vi "EditorEinfachCRIOalteMethoden-15-07-17.vi"() -> ()   [LabVIEW 2017]
panel:
  out "Methoden":T1(array[cluster])
  in  "Tab Control":T2(tab)
  in  "Dateiordner Housekeeping":path=path "C:/Users/Atmos/Desktop/Johnny"
  in  "Dateiname Housekeeping":string
  in  "DateiordnerECD1":path
  in  "DateinameECD1":string
  in  "DateiordnerECD2":path
  in  "DateinameECD2":string
  in  "Modul1/AI sicherer Bereich":dbl[][](array[numeric])=[[0.0, 0.0, 0.0, 0.0, 0.0, 0.0, 0.0, 0.0, 0.0, 0.0, 0.0, 0.0, 0.0, 0.0, 0.0, 0.0, 0.0, 0.0, 0.0, 0.0, 0.0, 0.0, 0.0, 0.0, 0.0, 0.0, 0.0, 0.0, 0.0, 0.0, 0.0, 0.0]]
  in  "Modul1/AIsNamen":string[](array[string])
  in  "Modul1/AI koeff":dbl[][](array[numeric])=[[0.0, 0.0, 0.0, 0.0, 0.0, 0.0, 0.0, 0.0, 0.0, 0.0, 0.0, 0.0, 0.0, 0.0, 0.0, 0.0, 0.0, 0.0, 0.0, 0.0, 0.0, 0.0, 0.0, 0.0, 0.0, 0.0, 0.0, 0.0, 0.0, 0.0, 0.0, 0.0]]
  in  "AIsNamenZurücksetzen":bool
  in  "Modul2/AIsNamen":string[](array[string])
  in  "Modul2/AI koeff":dbl[][](array[numeric])=[[0.0, 0.0, 0.0, 0.0, 0.0, 0.0, 0.0, 0.0, 0.0, 0.0, 0.0, 0.0, 0.0, 0.0, 0.0, 0.0, 0.0, 0.0, 0.0, 0.0, 0.0, 0.0, 0.0, 0.0, 0.0, 0.0, 0.0, 0.0, 0.0, 0.0, 0.0, 0.0]]
  in  "Modul2/AI sicherer Bereich":dbl[][](array[numeric])=[[0.0, 0.0, 0.0, 0.0, 0.0, 0.0, 0.0, 0.0, 0.0, 0.0, 0.0, 0.0, 0.0, 0.0, 0.0, 0.0, 0.0, 0.0, 0.0, 0.0, 0.0, 0.0, 0.0, 0.0, 0.0, 0.0, 0.0, 0.0, 0.0, 0.0, 0.0, 0.0]]
  in  "Modul3/AIsNamen":string[](array[string])
  in  "Modul3/AI koeff":dbl[][](array[numeric])=[[0.0, 0.0, 0.0, 0.0, 0.0, 0.0, 0.0, 0.0, 0.0, 0.0, 0.0, 0.0, 0.0, 0.0, 0.0, 0.0, 0.0, 0.0, 0.0, 0.0, 0.0, 0.0, 0.0, 0.0, 0.0, 0.0, 0.0, 0.0, 0.0, 0.0, 0.0, 0.0]]
  in  "Modul3/AI sicherer Bereich":dbl[][](array[numeric])=[[0.0, 0.0, 0.0, 0.0, 0.0, 0.0, 0.0, 0.0, 0.0, 0.0, 0.0, 0.0, 0.0, 0.0, 0.0, 0.0, 0.0, 0.0, 0.0, 0.0, 0.0, 0.0, 0.0, 0.0, 0.0, 0.0, 0.0, 0.0, 0.0, 0.0, 0.0, 0.0]]
  in  "Traps/MachsKoeff R(U)":dbl[][](array[numeric])=[[0.0, 0.0, 0.0, 0.0, 0.0, 0.0, 0.0, 0.0, 0.0, 0.0, 0.0, 0.0, 0.0, 0.0, 0.0, 0.0, 0.0, 0.0, 0.0, 0.0, 0.0, 0.0, 0.0, 0.0, 0.0, 0.0, 0.0, 0.0, 0.0, 0.0, 0.0, 0.0]]
  out "Schnelle Heizungen":string[](array[string])
  in  "Traps/MachsKoeff T(R)":dbl[][](array[numeric])=[[0.0, 0.0, 0.0, 0.0, 0.0, 0.0, 0.0, 0.0, 0.0, 0.0, 0.0, 0.0, 0.0, 0.0, 0.0, 0.0, 0.0, 0.0, 0.0, 0.0, 0.0, 0.0, 0.0, 0.0, 0.0, 0.0, 0.0, 0.0, 0.0, 0.0, 0.0, 0.0]]
  in  "Traps/Machs sicherer Bereich":dbl[][](array[numeric])=[[0.0, 0.0, 0.0, 0.0, 0.0, 0.0, 0.0, 0.0, 0.0, 0.0, 0.0, 0.0, 0.0, 0.0, 0.0, 0.0, 0.0, 0.0, 0.0, 0.0, 0.0, 0.0, 0.0, 0.0, 0.0, 0.0, 0.0, 0.0, 0.0, 0.0, 0.0, 0.0]]
  in  "LangsameHeizungen":string[](array[string])
  in  "ModuleLH":i32[](array[numeric]) min=1 max=3 step=1
  in  "AIsLH":i32[](array[numeric]) min=0 max=31 step=1
  in  "LHGruppe":bool[](array[boolean])
  in  "DIOsMod0Name":string[](array[string])
  in  "DIOsMod0Nr":i32[](array[numeric]) min=0 max=63 step=1
  in  "DIOsMod1Name":string[](array[string])
  in  "DIOsMod1Nr":i32[](array[numeric]) min=0 max=63 step=1
  in  "DIOsMod2AName":string[](array[string])
  in  "DIOsMod2ANr":i32[](array[numeric]) min=0 max=63 step=1
  in  "DIOsMod2BName":string[](array[string])
  in  "DIOsMod2BNr":i32[](array[numeric]) min=0 max=63 step=1
  out "AnzahlRegler/Modul":i32[](array[numeric])
  in  "Regler für den Probenfluß":i32
  in  "ReglerNameMod0":string[](array[string])
  in  "ReglerNameMod1":string[](array[string])
  in  "ReglerNameMod2A":string[](array[string])
  in  "ReglerNameMod2B":string[](array[string])
  in  "MWabfragenMod0":string[](array[string])=[":060F0401210120", ":06100401210120", ":06110401210120"]
  in  "MWabfragenMod1":string[](array[string])=[":060F0401210120", ":06100401210120", ":06110401210120"]
  in  "MWabfragenMod2A":string[](array[string])=[":060F0401210120", ":06100401210120", ":06110401210120"]
  in  "MWabfragenMod2B":string[](array[string])=[":060F0401210120", ":06100401210120", ":06110401210120"]
  in  "SPvorgebenMod0":string[](array[string])=[":060F020121", ":0610020121", ":0611020121"]
  in  "SPvorgebenMod1":string[](array[string])=[":060F020121", ":0610020121", ":0611020121"]
  in  "SPvorgebenMod2A":string[](array[string])=[":060F020121", ":0610020121", ":0611020121"]
  in  "SPvorgebenMod2B":string[](array[string])=[":060F020121", ":0610020121", ":0611020121"]
  in  "FaktorMod0":dbl[](array[numeric])=[9.375e-05, 9.375e-05, 9.375e-05]
  in  "FaktorMod1":dbl[](array[numeric])=[9.375e-05, 9.375e-05, 9.375e-05]
  in  "FaktorMod2A":dbl[](array[numeric])=[9.375e-05, 9.375e-05, 9.375e-05]
  in  "FaktorMod2B":dbl[](array[numeric])=[9.375e-05, 9.375e-05, 9.375e-05]
  in  "MWAntwortMod0":string[](array[string])=[":060F020121", ":0610020121", ":0611020121"]
  in  "MWAntwortMod1":string[](array[string])=[":060F020121", ":0610020121", ":0611020121"]
  in  "MWAntwortMod2A":string[](array[string])=[":060F020121", ":0610020121", ":0611020121"]
  in  "MWAntwortMod2B":string[](array[string])=[":060F020121", ":0610020121", ":0611020121"]
  in  "ReglerMod0 sicherer Bereich":dbl[][](array[numeric])=[[9.375e-05, 9.375e-05, 9.375e-05]]
  in  "ReglerMod1 sicherer Bereich":dbl[][](array[numeric])=[[9.375e-05, 9.375e-05, 9.375e-05]]
  in  "ReglerMod2A sicherer Bereich":dbl[][](array[numeric])=[[9.375e-05, 9.375e-05, 9.375e-05]]
  in  "ReglerMod2B sicherer Bereich":dbl[][](array[numeric])=[[9.375e-05, 9.375e-05, 9.375e-05]]
  in  "Metavariablen grüner Bereich":dbl[][](array[numeric])=[[0.0, 0.0, 0.0, 0.0, 0.0, 0.0, 0.0, 0.0, 0.0, 0.0, 0.0, 0.0, 0.0, 0.0, 0.0, 0.0, 0.0, 0.0, 0.0, 0.0, 0.0, 0.0, 0.0, 0.0, 0.0, 0.0, 0.0, 0.0, 0.0, 0.0, 0.0, 0.0]]
  in  "Metavariablen":string[](array[string])
  in  "Startmethode":i32=1
  in  "MethodeLöschen":bool
  in  "MethodeDuplizieren":bool
  in  "T_MainMach2":dbl[](array[numeric])
  in  "t_MainMach2":dbl[](array[numeric])
  in  "T_MainMach1":dbl[](array[numeric])
  in  "t_MainMach1":dbl[](array[numeric])
  in  "EinstellungenSpeichern":bool
  out "LangsameHeizungen":string[](array[string])
  in  "AllesSpeichern":bool
  in  "Methodenname":string
  in  "Int.Stop2":dbl
  in  "Int.Start2":dbl
  in  "Int.Stop1":dbl
  in  "Int.Start1":dbl
  in  "ZeitpktMS-2":dbl
  in  "ZeitpktMS-1":dbl
  in  "SPMPV":i32[](array[numeric])
  in  "ZeitpunkteMPV":dbl[](array[numeric])
  in  "Wert2":dbl
  in  "Vergleichsoperator2":dbl(ring) items=["<", "<=", "=", ">=", ">", "=/="]
  in  "AbfragbareVariablen2":dbl(ring) items=["T1-Trap1 [°C]", "T1-Trap2 [°C]", "T1-StirlingKühlkopf [°C]", "T1-PreCol1 [°C]", "T1-PreCol2 [°C]", "T1-MainCol1a [°C]", "T1-MainCol1b [°C]", "T1-MainCol2a [°C]", "T1-MainCol2b [°C]", "T1-Bronkhorst1a [°C]", "T1-Bronkhorst1b [°C]", "T1-Bronkhorst2a [°C]", "T1-Bronkhorst2b [°C]", "T1-2Pos1B [°C]", "T1-Spare9", "T1-2Pos1A [°C]", "T1-Spare10", "T1-TurboPump [°C]", "T1-StirlingPlatine [°C]", "T1-Spare5", "T1-Spare6", "T1-Spare7", "T1-Spare8", "F1-MFM1", "F1-MFM0D [mL]", "P1-HeliumHP [bara]", "P1-HeliumLP [bara]", "P1-PumpVordruck [mbara]", "TurboSpeed", "I1-MS-AC [A]", "I1-Trap1 [A]", "I1-Trap2 [A]", "T2-ECD1a", "T2-ECD1b", "T2-ECD2a", "T2-ECD2b", "T2-Col1a", "T2-Col1b", "T2-Col2a", "T2-Col2b", "T2-Spare1", "T2-Spare2", "T2-Oven_a", "T2-Oven_b", "T2-Spare3", "T2-Spare4", "T2-Spare5", "F2-MFM0", "F2-MFM2A", "F2-MFM2B", "P2-N2O_HP", "P2-N2O_LP", "P2-CO2_HP", "P2-CO2_LP", "AI-Spare1", "FL-MFM1000mL", "AI-Spare3", "AI-Spare4", "StirlingAlarm", "StirlingEmerg.", "AI-Spare7", "AI-Spare8", "AI-Spare9", "FL-MFM30mL", "T0-DC/DC5", "I0-24V_M0", "I0-48V_M1", "I0-24V_M1", "I0-28V_M2", "T0-Spare3", "T0-Spare2", "T0-Spare4", "T0-DC/DC7", "I0-20V_Laptop", "I0-28V_M1", "I0-24V_M2", "I0-12V_Licor", "T0-Spare1", "T0-Drier", "T0-Spare5", "F0-MFM0A [L]", "TL-Licor_a", "P0-Span-HP", "P0-spare1", "P0-Stickstoff-LP", "P0-Helium-LP", "P0-Cal-HP", "P0-P9Tavco[bar]", "F0-MFM0B [L]", "TL-Licor_b", "P0-Span-LP", "P0-spare2", "P0-Stickstoff-HP", "P0-Helium-HP", "P0-Cal-LP", "F0-MFM3", "T-Trap1", "T-Trap2", "T-PreMach1", "T-PreMach2", "T-MainMach1", "T-MainMach2", "PrC0 [bara]", "PrC0-Licor [bara]", "PrC1-Säule1 [bara]", "PrC1-Säule2 [bara]", "MFC1-Sample [ml/min]", "PrC1-BackFlush1 [bara]", "PrC1-BackFlush2 [bara]", "MFC1-Reaktant [l/min]", "MFC2A[ml/min]", "MFC2B[ml/min]", "MFC2C[ul/min]", "PrC2A[bara]", "MFC2D[ml/min]", "MFC2E[ml/min]", "PrC2B[bara]", "Gesamte Zeit", "Methodenzeit", "Zykluszeit Mod0", "Zykluszeit Mod1", "Zykluszeit Mod2A", "Zykluszeit Mod2B", "PositionMPV", "OverflowB", "OverflowA", "StirlingAlarmAlarm!"]
  in  "Dateien fürs MS schicken?":bool
  in  "Zwangsbedingungen":dbl[][](array[numeric])
  out "ZwangsBedingungen":string[][](array[string])
  in  "löschen":bool
  in  "Bedingung Nr. X":i32
  in  "Bedingung übernehmen":bool
  in  "Ausgangswert":dbl
  in  "BedienbareVariablen":dbl(ring) items=["D0-48V_M1", "D0-28V_M1", "D0-Pump2", "DL-LiCalS1H", "D-Spare2", "D-Spare4", "D0-28V_M2", "D0-Pump1", "D0-S01/EV1", "DL-Licor", "D0-EV3", "D0-EV2", "D1-StopMS", "D1-StartMS", "D1-TrapEvac1", "D1-TrapEvac2", "D1-2Pos1A", "D1-2Pos1B", "D1-TurboPump", "D1-PrePump", "D1-VacPump1", "D1-VacPump2", "D1-Stirling", "D1-P_MS", "D1-S1B(7)", "D1-S1A(6)", "D1-S1G", "D1-Fan3", "D1-LüfterMach1", "D1-LüfterMach2", "D1-MS-Power", "D2-SpülflußA", "D2-2Pos2A", "D2-Probe2A", "D2-ECD1HeaterOff", "D2-Fan1", "D2-Fan2", "D2-Spülfluß2B", "D2-2Pos2B", "D2-Probe2B", "D2-ECD2HeaterOff", "Heizen?Trap1", "Heizen?Trap2", "Heizen?PreMach1", "Heizen?PreMach2", "Heizen?MainMach1", "Heizen?MainMach2", "Methodennummer", "STOPP!!!", "H1-Valve1B heizen?", "H1-Bronkhorst1 heizen?", "H1-Bronkhorst2 heizen?", "H1-Valve1A heizen?", "H0-Drier heizen?", "HL-Licor heizen?", "H2-ECD2 heizen?", "H2-Oven heizen?", "H2-Spare1 heizen?", "H2-Col2 heizen?", "H2-Col1 heizen?", "H2-ECD1 heizen?", "PrC0 [bara]", "PrC0-Licor [bara]", "PrC1-Säule1 [bara]", "PrC1-Säule2 [bara]", "MFC1-Sample [ml/min]", "PrC1-BackFlush1 [bara]", "PrC1-BackFlush2 [bara]", "MFC1-Reaktant [l/min]", "MFC2A[ml/min]", "MFC2B[ml/min]", "MFC2C[ul/min]", "PrC2A[bara]", "MFC2D[ml/min]", "MFC2E[ml/min]", "PrC2B[bara]", "PositionMPV", "OverflowB", "OverflowA", "StirlingAlarmAlarm!"]
  in  "Wert1":dbl
  in  "Vergleichsoperator1":dbl(ring) items=["<", "<=", "=", ">=", ">", "=/="]
  in  "AbfragbareVariablen1":dbl(ring) items=["T1-Trap1 [°C]", "T1-Trap2 [°C]", "T1-StirlingKühlkopf [°C]", "T1-PreCol1 [°C]", "T1-PreCol2 [°C]", "T1-MainCol1a [°C]", "T1-MainCol1b [°C]", "T1-MainCol2a [°C]", "T1-MainCol2b [°C]", "T1-Bronkhorst1a [°C]", "T1-Bronkhorst1b [°C]", "T1-Bronkhorst2a [°C]", "T1-Bronkhorst2b [°C]", "T1-2Pos1B [°C]", "T1-Spare9", "T1-2Pos1A [°C]", "T1-Spare10", "T1-TurboPump [°C]", "T1-StirlingPlatine [°C]", "T1-Spare5", "T1-Spare6", "T1-Spare7", "T1-Spare8", "F1-MFM1", "F1-MFM0D [mL]", "P1-HeliumHP [bara]", "P1-HeliumLP [bara]", "P1-PumpVordruck [mbara]", "TurboSpeed", "I1-MS-AC [A]", "I1-Trap1 [A]", "I1-Trap2 [A]", "T2-ECD1a", "T2-ECD1b", "T2-ECD2a", "T2-ECD2b", "T2-Col1a", "T2-Col1b", "T2-Col2a", "T2-Col2b", "T2-Spare1", "T2-Spare2", "T2-Oven_a", "T2-Oven_b", "T2-Spare3", "T2-Spare4", "T2-Spare5", "F2-MFM0", "F2-MFM2A", "F2-MFM2B", "P2-N2O_HP", "P2-N2O_LP", "P2-CO2_HP", "P2-CO2_LP", "AI-Spare1", "FL-MFM1000mL", "AI-Spare3", "AI-Spare4", "StirlingAlarm", "StirlingEmerg.", "AI-Spare7", "AI-Spare8", "AI-Spare9", "FL-MFM30mL", "T0-DC/DC5", "I0-24V_M0", "I0-48V_M1", "I0-24V_M1", "I0-28V_M2", "T0-Spare3", "T0-Spare2", "T0-Spare4", "T0-DC/DC7", "I0-20V_Laptop", "I0-28V_M1", "I0-24V_M2", "I0-12V_Licor", "T0-Spare1", "T0-Drier", "T0-Spare5", "F0-MFM0A [L]", "TL-Licor_a", "P0-Span-HP", "P0-spare1", "P0-Stickstoff-LP", "P0-Helium-LP", "P0-Cal-HP", "P0-P9Tavco[bar]", "F0-MFM0B [L]", "TL-Licor_b", "P0-Span-LP", "P0-spare2", "P0-Stickstoff-HP", "P0-Helium-HP", "P0-Cal-LP", "F0-MFM3", "T-Trap1", "T-Trap2", "T-PreMach1", "T-PreMach2", "T-MainMach1", "T-MainMach2", "PrC0 [bara]", "PrC0-Licor [bara]", "PrC1-Säule1 [bara]", "PrC1-Säule2 [bara]", "MFC1-Sample [ml/min]", "PrC1-BackFlush1 [bara]", "PrC1-BackFlush2 [bara]", "MFC1-Reaktant [l/min]", "MFC2A[ml/min]", "MFC2B[ml/min]", "MFC2C[ul/min]", "PrC2A[bara]", "MFC2D[ml/min]", "MFC2E[ml/min]", "PrC2B[bara]", "Gesamte Zeit", "Methodenzeit", "Zykluszeit Mod0", "Zykluszeit Mod1", "Zykluszeit Mod2A", "Zykluszeit Mod2B", "PositionMPV", "OverflowB", "OverflowA", "StirlingAlarmAlarm!"]
  in  "Methode Nummer":i32
  in  "MethodeLaden":bool
  in  "EditorBeenden":bool
  in  "PIDs für \"träge\" Heizungen":T3(array[cluster])
  in  "T_PreMach2":dbl[](array[numeric])
  in  "t_PreMach2":dbl[](array[numeric])
  in  "T_PreMach1":dbl[](array[numeric])
  in  "t_PreMach1":dbl[](array[numeric])
  in  "SHSetpoints":dbl[][](array[numeric])
  in  "ZeitpktFPGAFixp":dbl[](array[numeric])
  in  "FPGAPID":T4(array[cluster])
  in  "ZeitpktFPGAPID":dbl[](array[numeric])
  in  "FPGABoolesch":bool[][](array[boolean])
  in  "ZPktFPGABoolesch":dbl[](array[numeric])
  in  "LHHeizen?":bool[](array[boolean])
  in  "LHSetpoints":dbl[](array[numeric])
  out "HorstMod1Name":string[](array[string])
  out "HorstMod2AName":string[](array[string])
  out "HorstMod2BName":string[](array[string])
  in  "HorstSPMod1":dbl[][](array[numeric])
  in  "HorstSPMod2A":dbl[][](array[numeric])
  in  "HorstSPMod2B":dbl[][](array[numeric])
  in  "Mod1HorstZeitpkt":dbl[](array[numeric])
  in  "Mod2AHorstZeitpkt":dbl[](array[numeric])
  in  "Mod2BHorstZeitpkt":dbl[](array[numeric])
  in  "HorstSPMod0":dbl[][](array[numeric])
  out "HorstMod0Name":string[](array[string])
  in  "Mod0HorstZeitpkt":dbl[](array[numeric])
  in  "DIOsSPMod2B":bool[][](array[boolean])
  in  "DIOsSPMod2A":bool[][](array[boolean])
  in  "DIOsSPMod1":bool[][](array[boolean])
  in  "ZeitpktDIOsMod2B":dbl[](array[numeric])
  in  "ZeitpktDIOsMod2A":dbl[](array[numeric])
  in  "ZeitpktDIOsMod1":dbl[](array[numeric])
  out "DIOsMod2BName":string[](array[string])
  out "DIOsMod2AName":string[](array[string])
  out "DIOsMod1Name":string[](array[string])
  out "DIOsMod0Name":string[](array[string])
  in  "DIOsSPMod0":bool[][](array[boolean])
  in  "ZeitpktDIOsMod0":dbl[](array[numeric])
  in  "MethodeSpeichern":bool
  in  "EinstellungenFertig":bool
  in  "Zykluslängen [s]":dbl[](array[numeric])
  # "Trap1          Trap2      PreMach1  PreMach2 MainMach1 MainMach2\n       heizen         heizen        heizen         heizen         heizen         heizen"
  # "Trap1"
  # "Trap2"
  # "PreMach1"
  # "PreMach2"
  # "MainMach1"
  # "MainMach2"
  # "Sososo... alle Einstellungen vorgenommen? Wirklich alle? Sicher? Bereit, mit den Methoden fortzufahren? Na super, dann trau Dich und drück den Knopf!"
  # "Es können beliebig viele Methoden definiert werden; die gewünschte Nummer auswählen und die entsprechende Methode laden, dann nach Belieben dran rumfummeln und anschließend, wenns beliebt, die vorgenommenen Änderungen an der Methode übernehmen (das bedeutet NICHT, daß die Änderungen in einer Datei abgelegt werden, dafür gibts nen extra Knopp);\n\"Editor beenden\" dürfte klar sein. Und Tschüß!"
  # ":::Tom \"Awesome\"  Burner Jr.:::"
  # "Sollen die Daten vom MS abgefragt werden? Wenn ja, zu welchen Zeitpunkten (im Zyklus1)?"
  # "Schnelle Heizungen..."
  # "Die eingegebenen Punkte im (t-T)-Raum werden durch lineare Funktionen verbunden, jeweils definiert von Punkt zu Punkt."
  # "Stellung des Multipositionsventils; die Zeitpunkte beziehen sich auf den Zyklus von Modul0.\nDie Stellungen bezeichnen: \n1. Cal - 2. Span - 3. ? - 4. ? - \n5. Plank - 6. Air - 7. ?"
  # "Innerhalb welcher Zeitfenster (Modul1) soll der Probenfluß integriert werden?"
  # "Der Gipfel der Flexibilität: die Zwangsbedingungen!\nBitte boolesche Werte als 0/1 eingeben"
  # "Mod0\n\nMod1\n\nMod2A\n\nMod2B"
  # "UND"
  # "TSetpTrap1                TSetpTrap2"
  # "Dran denken: die Daten werden auf dem CRIO abgelegt, nicht auf dem ITX oder dem Notebook; Dateinamen bitte ohne Pfad und .tdms eingeben!"
  # "Die Analogeingänge sind entsprechend der AI-Module des CRIO angeordnet (3x32); es wird eine quadratische Kennlinie angenommen, also: y=a0+a1*x+a2*x^2;\ndie drei Koeffizienten werden in dieser Reihenfolge eingegeben (v.l.n.r.): a0, a1, a2. Die Alarmgrenzen werden folgendermaßen eingegeben: linke Spalte für untere Grenze, rechte Spalte für obere Grenze des sicheren Bereichs."
  # "Die Analogeingänge sind entsprechend der AI-Module des CRIO angeordnet (3x32); es wird eine quadratische Kennlinie angenommen, also: y=a0+a1*x+a2*x^2;\ndie drei Koeffizienten werden in dieser Reihenfolge eingegeben (v.l.n.r.): a0, a1, a2. Die Alarmgrenzen werden folgendermaßen eingegeben: linke Spalte für untere Grenze, rechte Spalte für obere Grenze des sicheren Bereichs."
  # "Die Analogeingänge sind entsprechend der AI-Module des CRIO angeordnet (3x32); es wird eine quadratische Kennlinie angenommen, also: y=a0+a1*x+a2*x^2;\ndie drei Koeffizienten werden in dieser Reihenfolge eingegeben (v.l.n.r.): a0, a1, a2. Die Alarmgrenzen werden folgendermaßen eingegeben: linke Spalte für untere Grenze, rechte Spalte für obere Grenze des sicheren Bereichs."
  # "Vorsicht!!! Wer hier nicht ganz genau weiß, was er tut, läßt bitte die Finger davon!\nDie Heizungen werden über den FPGA gesteuert, d.h. wenn man die Anzahl oder die Anschlüsse der Heizungen ändert, muß das FPGA-Programm entsprechend angepaßt werden.\nModuleLH bezieht sich auf die drei AI-Module des CRIO (1,2,3) und AIsLH auf den Anschluß im jeweiligen Modul."
  # "Die digitalen Ein-/Ausgänge werden modulweise aufgelistet (0, 1, 2A, 2B) und benannt; die zugehörigen Anschlüsse werden folgendermaßen durchgezählt: \nDIO 0...31 von Modul5 entspricht hier 0...31; DIO 0...31 von Modul6 entspricht hier 32+(0...31)=32...63."
  # "Die Bronkhorst-Regler werden modulweise zusammengefasst an den CRIO angeschlossen, Mod0 an Port0, Mod1 an Port1, Mod2A&2B an Port2;\ndie Strings für die Steuerung und Abfrage der Regler ergeben sich aus dem bronkhorstschen Handbuch; der Faktor berechnet sich durch \"Vollausschlag des Reglers (in der gewünschten Einheit, z.B. Bar)\"/32000;\n'Regler für den Probenfluß' meint die Nummer des entsprechenden Reglers in der Liste aller Regler, wobei der erste die Nummer 0 trägt."
  # "Wer will noch mehr, wer hat noch nichts? An dieser Stelle können weitere Variablen definiert werden, mit deren Hilfe die Zwangsbedingungen erst ihre volle Pracht und Mächtigkeit entfalten. Alle Variablen sind numerische Größen und haben damit beliebig viele Zustände. Beim Programmstart werden sie mit Null initialisiert.\nHöchschte Vorsicht ist beim Umbenennen oder gar Löschen von Variablen geboten, weil sich das fatal auf bestehende Zwangsbedingungen auswirken kann. Am besten immer nur neue Variablen hinzufügen, das garantiert sicheren Spaß ohne Spätfolgen."
  # "Im weiteren können beliebig viele Methoden definiert werden; mit welcher davon soll das Programm starten? Die erste Methode trägt die Nummer 0."
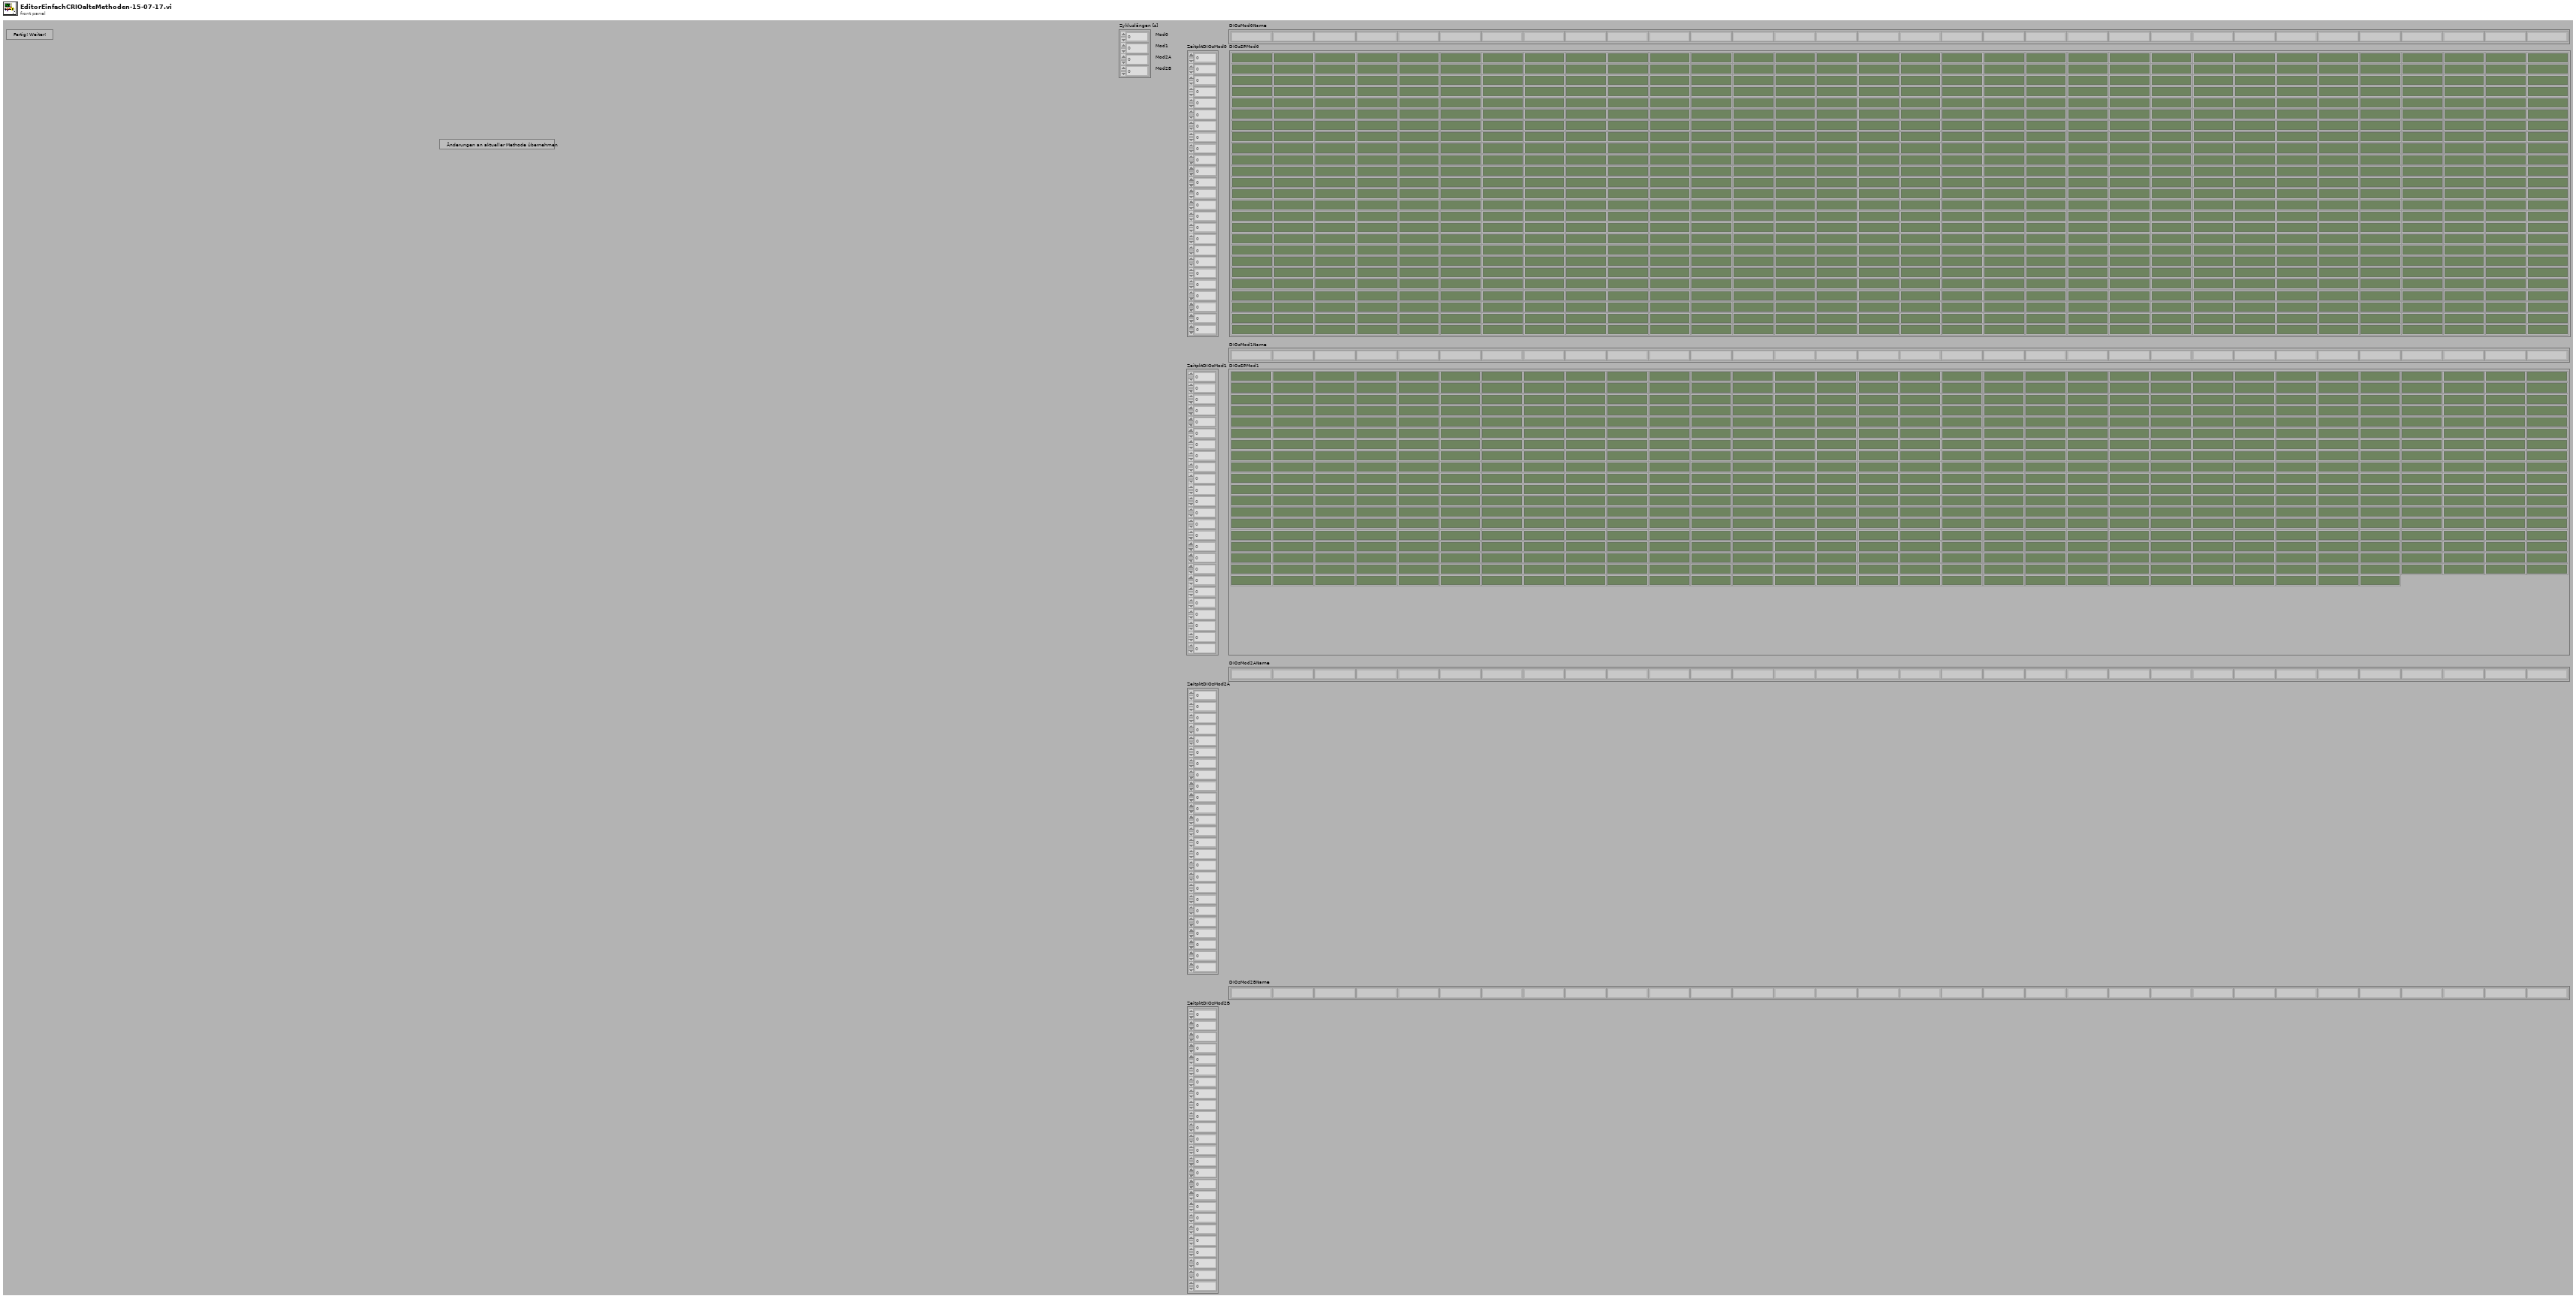
[diagram p1: front panel]
types:
  T1 = cluster{"Zykluslängen [s]":dbl[], "ZeitpktDIOsMod0":dbl[], "ZeitpktDIOsMod1":dbl[], "ZeitpktDIOsMod2A":dbl[], "ZeitpktDIOsMod2B":dbl[], "DIOsSPMod0":bool[][], "DIOsSPMod1":bool[][], "DIOsSPMod2A":bool[][], "DIOsSPMod2B":bool[][], "Mod0HorstZeitpkt":dbl[], "Mod1HorstZeitpkt":dbl[], "Mod2AHorstZeitpkt":dbl[], "Mod2BHorstZeitpkt":dbl[], "HorstSPMod0":dbl[][], "HorstSPMod1":dbl[][], "HorstSPMod2A":dbl[][], "HorstSPMod2B":dbl[][], "LHSetpoints":dbl[], "LHHeizen?":bool[], "ZPktFPGABoolesch":dbl[], "FPGABoolesch":bool[][], "ZeitpktFPGAPID":dbl[], "FPGAPID":cluster{"d0":fxp<+/-,18,18>, "d1":fxp<+/-,21,21>}[][], "ZeitpktFPGAFixp":dbl[], "SHSetpoints":dbl[][], "t_PreMach1":dbl[], "T_PreMach1":dbl[], "t_PreMach2":dbl[], "T_PreMach2":dbl[], "PIDs für \"träge\" Heizungen":cluster{"proportional gain (Kc)":dbl, "integral time (Ti, min)":dbl, "derivative time (Td, min)":dbl}[], "Zwangsbedingungen":dbl[][], "Dateien fürs MS schicken?":bool, "ZeitpunkteMPV":dbl[], "SPMPV":i32[], "ZeitpktMS-1":dbl, "ZeitpktMS-2":dbl, "Int.Start1":dbl, "Int.Stop1":dbl, "Int.Start2":dbl, "Int.Stop2":dbl, "Methodenname":string, "t_MainMach1":dbl[], "T_MainMach1":dbl[], "t_MainMach2":dbl[], "T_MainMach2":dbl[]}[]
  T2 = enum32{"Dateinamen", "Modul1/AIs", "Modul2/AIs", "Modul3/AIs", "schnelle Heizungen", "langsame Heizungen", "DIOs", "Horst-Regler", "Metavariablen", "Startmethode"}
  T3 = cluster{"proportional gain":dbl, "integral time":dbl, "derivative time":dbl}[]
  T4 = cluster{"d0":fxp<+/-,18,18>, "d1":fxp<+/-,21,21>}[][]
  T5 = cluster{"DIOsMod0Nr":i32[], "DIOsMod1Nr":i32[], "DIOsMod2ANr":i32[], "DIOsMod2BNr":i32[], "AIsLH":i32[], "AnzahlRegler/Modul":i32[], "Regler für den Probenfluß":i32, "SPvorgebenMod0":string[], "SPvorgebenMod1":string[], "SPvorgebenMod2A":string[], "SPvorgebenMod2B":string[], "MWAntwortMod0":string[], "MWAntwortMod1":string[], "MWAntwortMod2A":string[], "MWAntwortMod2B":string[], "FaktorMod0":dbl[], "FaktorMod1":dbl[], "FaktorMod2A":dbl[], "FaktorMod2B":dbl[], "MWabfragenMod0":string[], "MWabfragenMod1":string[], "MWabfragenMod2A":string[], "MWabfragenMod2B":string[], "Modul1/AI koeff":dbl[][], "Modul2/AI koeff":dbl[][], "Modul3/AI koeff":dbl[][], "Traps/MachsKoeff":dbl[][], "Modul1/AIsNamen":string[], "Modul2/AIsNamen":string[], "Modul3/AIsNamen":string[], "DIOsMod0Name":string[], "DIOsMod1Name":string[], "DIOsMod2AName":string[], "DIOsMod2BName":string[], "ReglerNameMod0":string[], "ReglerNameMod1":string[], "ReglerNameMod2A":string[], "ReglerNameMod2B":string[], "Startmethode":i32, "Dateiordner Housekeeping":path, "Dateiname Housekeeping":string, "DateiordnerECD1":path, "DateinameECD1":string, "DateiordnerECD2":path, "DateinameECD2":string, "LangsameHeizungen":string[], "ModuleLH":i32[], "Metavariablen":string[], "Modul1/AI sicherer Bereich":dbl[][], "Modul2/AI sicherer Bereich":dbl[][], "Modul3/AI sicherer Bereich":dbl[][], "Traps/Machs sicherer Bereich":dbl[][], "ReglerMod0 sicherer Bereich":dbl[][], "ReglerMod1 sicherer Bereich":dbl[][], "ReglerMod2A sicherer Bereich":dbl[][], "ReglerMod2B sicherer Bereich":dbl[][], "Metavariablen grüner Bereich":dbl[][]}
  T6 = cluster{"Zykluslängen [s]":dbl[], "ZeitpktDIOsMod0":dbl[], "ZeitpktDIOsMod1":dbl[], "ZeitpktDIOsMod2A":dbl[], "ZeitpktDIOsMod2B":dbl[], "DIOsSPMod0":bool[][], "DIOsSPMod1":bool[][], "DIOsSPMod2A":bool[][], "DIOsSPMod2B":bool[][], "Mod0HorstZeitpkt":dbl[], "Mod1HorstZeitpkt":dbl[], "Mod2AHorstZeitpkt":dbl[], "Mod2BHorstZeitpkt":dbl[], "HorstSPMod0":dbl[][], "HorstSPMod1":dbl[][], "HorstSPMod2A":dbl[][], "HorstSPMod2B":dbl[][], "LHSetpoints":dbl[], "LHHeizen?":bool[], "ZPktFPGABoolesch":dbl[], "FPGABoolesch":bool[][], "ZeitpktFPGAPID":dbl[], "FPGAPID":cluster{"proportional gain (Kc)":fxp<+/-,16,8>, "integral gain (Kc*Ts/Ti)":fxp<+/-,16,8>, "derivative gain (Kc*Td/Ts)":fxp<+/-,16,8>}[][], "ZeitpktFPGAFixp":dbl[], "SHSetpoints":dbl[][], "t_PreMach1":dbl[], "T_PreMach1":dbl[], "t_PreMach2":dbl[], "T_PreMach2":dbl[], "PIDs für \"träge\" Heizungen":cluster{"proportional gain (Kc)":dbl, "integral time (Ti, min)":dbl, "derivative time (Td, min)":dbl}[], "Zwangsbedingungen":dbl[][], "Dateien fürs MS schicken?":bool, "ZeitpunkteMPV":dbl[], "SPMPV":i32[], "ZeitpktMS-1":dbl, "ZeitpktMS-2":dbl, "Int.Start1":dbl, "Int.Stop1":dbl, "Int.Start2":dbl, "Int.Stop2":dbl, "Methodenname":string, "t_MainMach1":dbl[], "T_MainMach1":dbl[], "t_MainMach2":dbl[], "T_MainMach2":dbl[]}[]
  T7 = enum16{"open", "replace", "create", "open or create", "replace or create", "replace or create with confirmation"}
  T8 = cluster{"DIOsMod0Nr":i32[], "DIOsMod1Nr":i32[], "DIOsMod2ANr":i32[], "DIOsMod2BNr":i32[], "AIsLH":i32[], "AnzahlRegler/Modul":i32[], "Regler für den Probenfluß":i32, "SPvorgebenMod0":string[], "SPvorgebenMod1":string[], "SPvorgebenMod2A":string[], "SPvorgebenMod2B":string[], "MWAntwortMod0":string[], "MWAntwortMod1":string[], "MWAntwortMod2A":string[], "MWAntwortMod2B":string[], "FaktorMod0":dbl[], "FaktorMod1":dbl[], "FaktorMod2A":dbl[], "FaktorMod2B":dbl[], "MWabfragenMod0":string[], "MWabfragenMod1":string[], "MWabfragenMod2A":string[], "MWabfragenMod2B":string[], "Modul1/AI koeff":dbl[][], "Modul2/AI koeff":dbl[][], "Modul3/AI koeff":dbl[][], "Traps/MachsKoeff T(R)":dbl[][], "Modul1/AIsNamen":string[], "Modul2/AIsNamen":string[], "Modul3/AIsNamen":string[], "DIOsMod0Name":string[], "DIOsMod1Name":string[], "DIOsMod2AName":string[], "DIOsMod2BName":string[], "ReglerNameMod0":string[], "ReglerNameMod1":string[], "ReglerNameMod2A":string[], "ReglerNameMod2B":string[], "Startmethode":i32, "Dateiordner Housekeeping":path, "Dateiname Housekeeping":string, "DateiordnerECD1":path, "DateinameECD1":string, "DateiordnerECD2":path, "DateinameECD2":string, "LangsameHeizungen":string[], "ModuleLH":i32[], "Metavariablen":string[], "Modul1/AI sicherer Bereich":dbl[][], "Modul2/AI sicherer Bereich":dbl[][], "Modul3/AI sicherer Bereich":dbl[][], "Traps/Machs sicherer Bereich":dbl[][], "ReglerMod0 sicherer Bereich":dbl[][], "ReglerMod1 sicherer Bereich":dbl[][], "ReglerMod2A sicherer Bereich":dbl[][], "ReglerMod2B sicherer Bereich":dbl[][], "Metavariablen grüner Bereich":dbl[][], "Traps/MachsKoeff R(U)":dbl[][], "LHGruppe":bool[]}
  T9 = cluster{"proportional gain (Kc)":dbl, "integral time (Ti, min)":dbl, "derivative time (Td, min)":dbl}[]
  T10 = cluster{"Zykluslängen [s]":dbl[], "ZeitpktDIOsMod0":dbl[], "ZeitpktDIOsMod1":dbl[], "ZeitpktDIOsMod2A":dbl[], "ZeitpktDIOsMod2B":dbl[], "DIOsSPMod0":bool[][], "DIOsSPMod1":bool[][], "DIOsSPMod2A":bool[][], "DIOsSPMod2B":bool[][], "Mod0HorstZeitpkt":dbl[], "Mod1HorstZeitpkt":dbl[], "Mod2AHorstZeitpkt":dbl[], "Mod2BHorstZeitpkt":dbl[], "HorstSPMod0":dbl[][], "HorstSPMod1":dbl[][], "HorstSPMod2A":dbl[][], "HorstSPMod2B":dbl[][], "LHSetpoints":dbl[], "LHHeizen?":bool[], "ZPktFPGABoolesch":dbl[], "FPGABoolesch":bool[][], "ZeitpktFPGAPID":dbl[], "FPGAPID":cluster{"d0":fxp<+/-,18,18>, "d1":fxp<+/-,21,21>}[][], "ZeitpktFPGAFixp":dbl[], dbl[][], "t_PreMach1":dbl[], "T_PreMach1":dbl[], "t_PreMach2":dbl[], "T_PreMach2":dbl[], "PIDs für \"träge\" Heizungen":cluster{"proportional gain (Kc)":dbl, "integral time (Ti, min)":dbl, "derivative time (Td, min)":dbl}[], "Zwangsbedingungen":dbl[][], "Dateien fürs MS schicken?":bool, "ZeitpunkteMPV":dbl[], "SPMPV":i32[], "ZeitpktMS-1":dbl, "ZeitpktMS-2":dbl, "Int.Start1":dbl, "Int.Stop1":dbl, "Int.Start2":dbl, "Int.Stop2":dbl, "Methodenname":string, "t_MainMach1":dbl[], "T_MainMach1":dbl[], "t_MainMach2":dbl[], "T_MainMach2":dbl[]}
  T11 = cluster{"Zykluslängen [s]":dbl[], "ZeitpktDIOsMod0":dbl[], "ZeitpktDIOsMod1":dbl[], "ZeitpktDIOsMod2A":dbl[], "ZeitpktDIOsMod2B":dbl[], "DIOsSPMod0":bool[][], "DIOsSPMod1":bool[][], "DIOsSPMod2A":bool[][], "DIOsSPMod2B":bool[][], "Mod0HorstZeitpkt":dbl[], "Mod1HorstZeitpkt":dbl[], "Mod2AHorstZeitpkt":dbl[], "Mod2BHorstZeitpkt":dbl[], "HorstSPMod0":dbl[][], "HorstSPMod1":dbl[][], "HorstSPMod2A":dbl[][], "HorstSPMod2B":dbl[][], "LHSetpoints":dbl[], "LHHeizen?":bool[], "ZPktFPGABoolesch":dbl[], "FPGABoolesch":bool[][], "ZeitpktFPGAPID":dbl[], "FPGAPID":cluster{"d0":fxp<+/-,18,18>, "d1":fxp<+/-,21,21>}[][], "ZeitpktFPGAFixp":dbl[], "SHSetpoints":dbl[][], "t_PreMach1":dbl[], "T_PreMach1":dbl[], "t_PreMach2":dbl[], "T_PreMach2":dbl[], "PIDs für \"träge\" Heizungen":cluster{"proportional gain":dbl, "integral time":dbl, "derivative time":dbl}[], "Zwangsbedingungen":dbl[][], "Dateien fürs MS schicken?":bool, "ZeitpunkteMPV":dbl[], "SPMPV":i32[], "ZeitpktMS-1":dbl, "ZeitpktMS-2":dbl, "Int.Start1":dbl, "Int.Stop1":dbl, "Int.Start2":dbl, "Int.Stop2":dbl, "Methodenname":string, "t_MainMach1":dbl[], "T_MainMach1":dbl[], "t_MainMach2":dbl[], "T_MainMach2":dbl[]}
  T12 = cluster{"Zykluslängen [s]":dbl[], "ZeitpktDIOsMod0":dbl[], "ZeitpktDIOsMod1":dbl[], "ZeitpktDIOsMod2A":dbl[], "ZeitpktDIOsMod2B":dbl[], "DIOsSPMod0":bool[][], "DIOsSPMod1":bool[][], "DIOsSPMod2A":bool[][], "DIOsSPMod2B":bool[][], "Mod0HorstZeitpkt":dbl[], "Mod1HorstZeitpkt":dbl[], "Mod2AHorstZeitpkt":dbl[], "Mod2BHorstZeitpkt":dbl[], "HorstSPMod0":dbl[][], "HorstSPMod1":dbl[][], "HorstSPMod2A":dbl[][], "HorstSPMod2B":dbl[][], "LHSetpoints":dbl[], "LHHeizen?":bool[], "ZPktFPGABoolesch":dbl[], "FPGABoolesch":bool[][], "ZeitpktFPGAPID":dbl[], "FPGAPID":cluster{"d0":fxp<+/-,18,18>, "d1":fxp<+/-,21,21>}[][], "ZeitpktFPGAFixp":dbl[], dbl[][], "t_PreMach1":dbl[], "T_PreMach1":dbl[], "t_PreMach2":dbl[], "T_PreMach2":dbl[], "PIDs für \"träge\" Heizungen":cluster{"proportional gain (Kc)":dbl, "integral time (Ti, min)":dbl, "derivative time (Td, min)":dbl}[], "Zwangsbedingungen":dbl[][], "Dateien fürs MS schicken?":bool, "ZeitpunkteMPV":dbl[], "SPMPV":i32[], "ZeitpktMS-1":dbl, "ZeitpktMS-2":dbl, "Int.Start1":dbl, "Int.Stop1":dbl, "Int.Start2":dbl, "Int.Stop2":dbl, "Methodenname":string, "t_MainMach1":dbl[], "T_MainMach1":dbl[], "t_MainMach2":dbl[], "T_MainMach2":dbl[]}[]
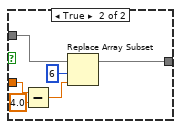
[diagram p4: hidden frame]
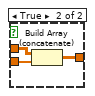
[diagram p10: hidden frame]
diagram:
  n1 = Open/Create/Replace File(file path (use dialog)=path "c:/einstellungen.perx" ("Dateipfad Einstellungen")) -> (refnum out=w23:refnum<file>, error out=w24:errorcluster)  [unwired: 5 in, 1 out]
  n2 = Read from Binary File(5:T5 {"DIOsMod0Nr"=[], "DIOsMod1Nr"=[], "DIOsMod2ANr"=[], "DIOsMod2BNr"=[], "AIsLH"=[], "AnzahlRegler/Modul"=[], "Regler für den Probenfluß"=0, "SPvorgebenMod0"=[], "SPvorgebenMod1"=[], "SPvorgebenMod2A"=[], "SPvorgebenMod2B"=[], "MWAntwortMod0"=[], "MWAntwortMod1"=[], "MWAntwortMod2A"=[], "MWAntwortMod2B"=[], "FaktorMod0"=[], "FaktorMod1"=[], "FaktorMod2A"=[], "FaktorMod2B"=[], "MWabfragenMod0"=[], "MWabfragenMod1"=[], "MWabfragenMod2A"=[], "MWabfragenMod2B"=[], "Modul1/AI koeff"=[], "Modul2/AI koeff"=[], "Modul3/AI koeff"=[], "Traps/MachsKoeff"=[], "Modul1/AIsNamen"=[], "Modul2/AIsNamen"=[], "Modul3/AIsNamen"=[], "DIOsMod0Name"=[], "DIOsMod1Name"=[], "DIOsMod2AName"=[], "DIOsMod2BName"=[], "ReglerNameMod0"=[], "ReglerNameMod1"=[], "ReglerNameMod2A"=[], "ReglerNameMod2B"=[], "Startmethode"=0, "Dateiordner Housekeeping"=path "", "Dateiname Housekeeping"="", "DateiordnerECD1"=path "", "DateinameECD1"="", "DateiordnerECD2"=path "", "DateinameECD2"="", "LangsameHeizungen"=[], "ModuleLH"=[], "Metavariablen"=[], "Modul1/AI sicherer Bereich"=[], "Modul2/AI sicherer Bereich"=[], "Modul3/AI sicherer Bereich"=[], "Traps/Machs sicherer Bereich"=[], "ReglerMod0 sicherer Bereich"=[], "ReglerMod1 sicherer Bereich"=[], "ReglerMod2A sicherer Bereich"=[], "ReglerMod2B sicherer Bereich"=[], "Metavariablen grüner Bereich"=[]} ("output cluster"), 8:w24, 11:w23) -> (0:w21:errorcluster, 2:w8:T5, 3:w22:refnum<file>)  [unwired: 3 in, 1 out]
  n3 = Close File(refnum=w22, error in=w21) -> (error out=w20:errorcluster)  [unwired: 1 out]
  n4 = flat-sequence {
    tunnel: w8 -> [w99]
    tunnel: [w52] -> w12
    tunnel: [w121] -> w40
    tunnel: [w120] -> w39
    tunnel: [w119] -> w38
    tunnel: [w118] -> w37
    tunnel: [w117] -> w36
    tunnel: [w116] -> w35
    tunnel: [w115] -> w34
    tunnel: [w114] -> w33
    tunnel: [w113] -> w32
    tunnel: [w108] -> w31
    tunnel: [w107] -> w30
    tunnel: [w106] -> w29
    tunnel: [w105] -> w28
    tunnel: [w104] -> w27
    tunnel: [w103] -> w26
    tunnel: [w102] -> w13
    tunnel: w12 -> [w102]
    tunnel: [w101] -> w10
    tunnel: [w100] -> w9
    tunnel: w40 -> [w242]
    tunnel: w39 -> [w241]
    tunnel: w38 -> [w240]
    tunnel: w37 -> [w239]
    tunnel: w36 -> [w238]
    tunnel: w35 -> [w237]
    tunnel: w34 -> [w235]
    tunnel: w33 -> [w236]
    tunnel: w32 -> [w234]
    tunnel: w31 -> [w221]
    tunnel: w30 -> [w232]
    tunnel: w29 -> [w231]
    tunnel: w28 -> [w230]
    tunnel: w27 -> [w229]
    tunnel: w26 -> [w224]
    tunnel: w1 -> [w223]
    tunnel: w13 -> [w220]
    tunnel: w10 -> [w218]
    tunnel: w9 -> [w216]
    tunnel: w6 -> [w212]
    frame #0 {
      n5 = Unbundle(w99) -> ("DIOsMod0Nr"=w98:i32[], "DIOsMod1Nr"=w97:i32[], "DIOsMod2ANr"=w96:i32[], "DIOsMod2BNr"=w95:i32[], "AIsLH"=w94:i32[], "AnzahlRegler/Modul"=w93:i32[], "Regler für den Probenfluß"=w92:i32, "SPvorgebenMod0"=w91:string[], "SPvorgebenMod1"=w90:string[], "SPvorgebenMod2A"=w89:string[], "SPvorgebenMod2B"=w88:string[], "MWAntwortMod0"=w87:string[], "MWAntwortMod1"=w86:string[], "MWAntwortMod2A"=w85:string[], "MWAntwortMod2B"=w84:string[], "FaktorMod0"=w83:dbl[], "FaktorMod1"=w82:dbl[], "FaktorMod2A"=w81:dbl[], "FaktorMod2B"=w80:dbl[], "MWabfragenMod0"=w79:string[], "MWabfragenMod1"=w78:string[], "MWabfragenMod2A"=w77:string[], "MWabfragenMod2B"=w76:string[], "Modul1/AI koeff"=w75:dbl[][], "Modul2/AI koeff"=w74:dbl[][], "Modul3/AI koeff"=w73:dbl[][], "Traps/MachsKoeff"=w72:dbl[][], "Modul1/AIsNamen"=w71:string[], "Modul2/AIsNamen"=w70:string[], "Modul3/AIsNamen"=w69:string[], "DIOsMod0Name"=w68:string[], "DIOsMod1Name"=w67:string[], "DIOsMod2AName"=w66:string[], "DIOsMod2BName"=w65:string[], "ReglerNameMod0"=w64:string[], "ReglerNameMod1"=w63:string[], "ReglerNameMod2A"=w62:string[], "ReglerNameMod2B"=w61:string[], "Startmethode"=w60:i32, "Dateiordner Housekeeping"=w50:path, "Dateiname Housekeeping"=w59:string, "DateiordnerECD1"=w58:path, "DateinameECD1"=w57:string, "DateiordnerECD2"=w56:path, "DateinameECD2"=w55:string, "LangsameHeizungen"=w52:string[], "ModuleLH"=w53:i32[], "Metavariablen"=w51:string[], "Modul1/AI sicherer Bereich"=w49:dbl[][], "Modul2/AI sicherer Bereich"=w48:dbl[][], "Modul3/AI sicherer Bereich"=w47:dbl[][], "Traps/Machs sicherer Bereich"=w46:dbl[][], "ReglerMod0 sicherer Bereich"=w45:dbl[][], "ReglerMod1 sicherer Bereich"=w44:dbl[][], "ReglerMod2A sicherer Bereich"=w43:dbl[][], "ReglerMod2B sicherer Bereich"=w42:dbl[][], "Metavariablen grüner Bereich"=w41:dbl[][])
      n6 = property on="Modul1/AI sicherer Bereich" class="Arr (strikt)"("Value"=w49) -> ()  [unwired: 2 in, 2 out]
      n7 = property on="Modul3/AI sicherer Bereich" class="Arr (strikt)"("Value"=w47) -> ()  [unwired: 2 in, 2 out]
      n8 = property on="ReglerMod0 sicherer Bereich" class="Arr (strikt)"("Value"=w45) -> ()  [unwired: 2 in, 2 out]
      n9 = property on="ReglerMod1 sicherer Bereich" class="Arr (strikt)"("Value"=w44) -> ()  [unwired: 2 in, 2 out]
      n10 = property on="Modul2/AI sicherer Bereich" class="Arr (strikt)"("Value"=w48) -> ()  [unwired: 2 in, 2 out]
      n11 = property on="Traps/Machs sicherer Bereich" class="Arr (strikt)"("Value"=w46) -> ()  [unwired: 2 in, 2 out]
      n12 = property on="ReglerMod2A sicherer Bereich" class="Arr (strikt)"("Value"=w43) -> ()  [unwired: 2 in, 2 out]
      n13 = property on="ReglerMod2B sicherer Bereich" class="Arr (strikt)"("Value"=w42) -> ()  [unwired: 2 in, 2 out]
      n14 = property on="Metavariablen grüner Bereich" class="Arr (strikt)"("Value"=w41) -> ()  [unwired: 2 in, 2 out]
      n15 = invoke on="MethodeLöschen" class="Bool (strict)" method="Std wiederherstellen"() -> ()  [unwired: 3 in, 3 out]
      n16 = property on="ModuleLH" class="Arr (strikt)"("Value"=w53) -> ()  [unwired: 2 in, 2 out]
      n17 = property on="AIsLH" class="Arr (strikt)"("Value"=w94) -> ()  [unwired: 2 in, 2 out]
      n18 = property on="Dateiname Housekeeping" class="Str"("Value"=w59) -> ()  [unwired: 2 in, 2 out]
      n19 = property on="DIOsMod0Nr" class="Arr (strikt)"("Value"=w98) -> ()  [unwired: 2 in, 2 out]
      n20 = property on="DateiordnerECD1" class="Pfad"("Value"=w58) -> ()  [unwired: 2 in, 2 out]
      n21 = property on="DIOsMod1Nr" class="Arr (strikt)"("Value"=w97) -> ()  [unwired: 2 in, 2 out]
      n22 = property on="DateinameECD1" class="Str"("Value"=w57) -> ()  [unwired: 2 in, 2 out]
      n23 = property on="DateiordnerECD2" class="Pfad"("Value"=w56) -> ()  [unwired: 2 in, 2 out]
      n24 = property on="DateinameECD2" class="Str"("Value"=w55) -> ()  [unwired: 2 in, 2 out]
      n25 = property on="DIOsMod2ANr" class="Arr (strikt)"("Value"=w96) -> ()  [unwired: 2 in, 2 out]
      n26 = property on="LangsameHeizungen" class="Arr (strikt)"("Value"=w52) -> ()  [unwired: 2 in, 2 out]
      n27 = property on="Metavariablen" class="Arr (strikt)"("Value"=w51) -> ()  [unwired: 2 in, 2 out]
      n28 = property on="DIOsMod2BNr" class="Arr (strikt)"("Value"=w95) -> ()  [unwired: 2 in, 2 out]
      n29 = property on="AnzahlRegler/Modul" class="Arr (strikt)"("Value"=w93) -> ()  [unwired: 2 in, 2 out]
      n30 = property on="Regler für den Probenfluß" class="DigWert (strikt)"("Value"=w92) -> ()  [unwired: 2 in, 2 out]
      n31 = property on="SPvorgebenMod0" class="Arr (strikt)"("Value"=w91) -> ()  [unwired: 2 in, 2 out]
      n32 = property on="ReglerNameMod2B" class="Arr (strikt)"("Value"=w61) -> ()  [unwired: 2 in, 2 out]
      n33 = property on="Startmethode" class="DigWert (strikt)"("Value"=w60) -> ()  [unwired: 2 in, 2 out]
      n34 = property on="Dateiordner Housekeeping" class="Pfad"("Value"=w50) -> ()  [unwired: 2 in, 2 out]
      n35 = property on="SPvorgebenMod1" class="Arr (strikt)"("Value"=w90) -> ()  [unwired: 2 in, 2 out]
      n36 = property on="SPvorgebenMod2A" class="Arr (strikt)"("Value"=w89) -> ()  [unwired: 2 in, 2 out]
      n37 = property on="SPvorgebenMod2B" class="Arr (strikt)"("Value"=w88) -> ()  [unwired: 2 in, 2 out]
      n38 = property on="MWAntwortMod0" class="Arr (strikt)"("Value"=w87) -> ()  [unwired: 2 in, 2 out]
      n39 = property on="MWAntwortMod1" class="Arr (strikt)"("Value"=w86) -> ()  [unwired: 2 in, 2 out]
      n40 = property on="MWAntwortMod2A" class="Arr (strikt)"("Value"=w85) -> ()  [unwired: 2 in, 2 out]
      n41 = property on="MWAntwortMod2B" class="Arr (strikt)"("Value"=w84) -> ()  [unwired: 2 in, 2 out]
      n42 = property on="FaktorMod0" class="Arr (strikt)"("Value"=w83) -> ()  [unwired: 2 in, 2 out]
      n43 = property on="FaktorMod1" class="Arr (strikt)"("Value"=w82) -> ()  [unwired: 2 in, 2 out]
      n44 = property on="FaktorMod2B" class="Arr (strikt)"("Value"=w80) -> ()  [unwired: 2 in, 2 out]
      n45 = property on="MWabfragenMod0" class="Arr (strikt)"("Value"=w79) -> ()  [unwired: 2 in, 2 out]
      n46 = property on="FaktorMod2A" class="Arr (strikt)"("Value"=w81) -> ()  [unwired: 2 in, 2 out]
      n47 = property on="MWabfragenMod1" class="Arr (strikt)"("Value"=w78) -> ()  [unwired: 2 in, 2 out]
      n48 = property on="MWabfragenMod2A" class="Arr (strikt)"("Value"=w77) -> ()  [unwired: 2 in, 2 out]
      n49 = property on="MWabfragenMod2B" class="Arr (strikt)"("Value"=w76) -> ()  [unwired: 2 in, 2 out]
      n50 = property on="Modul1/AI koeff" class="Arr (strikt)"("Value"=w75) -> ()  [unwired: 2 in, 2 out]
      n51 = property on="Modul3/AI koeff" class="Arr (strikt)"("Value"=w73) -> ()  [unwired: 2 in, 2 out]
      n52 = property on="Traps/MachsKoeff T(R)" class="Arr (strikt)"("Value"=w72) -> ()  [unwired: 2 in, 2 out]
      n53 = property on="Modul1/AIsNamen" class="Arr (strikt)"("Value"=w71) -> ()  [unwired: 2 in, 2 out]
      n54 = property on="Modul2/AIsNamen" class="Arr (strikt)"("Value"=w70) -> ()  [unwired: 2 in, 2 out]
      n55 = property on="Modul3/AIsNamen" class="Arr (strikt)"("Value"=w69) -> ()  [unwired: 2 in, 2 out]
      n56 = property on="Modul2/AI koeff" class="Arr (strikt)"("Value"=w74) -> ()  [unwired: 2 in, 2 out]
      n57 = property on="DIOsMod0Name" class="Arr (strikt)"("Value"=w68) -> ()  [unwired: 2 in, 2 out]
      n58 = property on="DIOsMod1Name" class="Arr (strikt)"("Value"=w67) -> ()  [unwired: 2 in, 2 out]
      n59 = property on="DIOsMod2AName" class="Arr (strikt)"("Value"=w66) -> ()  [unwired: 2 in, 2 out]
      n60 = property on="DIOsMod2BName" class="Arr (strikt)"("Value"=w65) -> ()  [unwired: 2 in, 2 out]
      n61 = property on="ReglerNameMod0" class="Arr (strikt)"("Value"=w64) -> ()  [unwired: 2 in, 2 out]
      n62 = property on="ReglerNameMod1" class="Arr (strikt)"("Value"=w63) -> ()  [unwired: 2 in, 2 out]
      n63 = property on="ReglerNameMod2A" class="Arr (strikt)"("Value"=w62) -> ()  [unwired: 2 in, 2 out]
      "Schnelle Heizungen" <- string[] ["Trap1 [°C]", "Trap2 [°C]", "PreCol1 [°C]", "PreCol2 [°C]", "MainCol1 [°C]", "MainCol2 [°C]"]
    }
    frame #1 {
      n64 = while {
        tunnel: ["DIOsMod0Name"] -> w121
        tunnel: ["DIOsMod1Name"] -> w120
        tunnel: ["DIOsMod2AName"] -> w119
        tunnel: ["DIOsMod2BName"] -> w118
        tunnel: ["ReglerNameMod0"] -> w117
        tunnel: ["ReglerNameMod1"] -> w116
        tunnel: ["ReglerNameMod2A"] -> w115
        tunnel: ["ReglerNameMod2B"] -> w114
        tunnel: [w140] -> w113
        tunnel: ["ReglerNameMod2B"] -> w112
        tunnel: ["ReglerNameMod2A"] -> w111
        tunnel: ["ReglerNameMod1"] -> w110
        tunnel: ["ReglerNameMod0"] -> w109
        tunnel: ["DIOsMod0Name"] -> w107
        tunnel: ["DIOsMod1Name"] -> w106
        tunnel: ["DIOsMod2AName"] -> w105
        tunnel: ["DIOsMod2BName"] -> w104
        tunnel: ["LangsameHeizungen"] -> w103
        tunnel: ["Metavariablen"] -> w101
        tunnel: ["Metavariablen"] -> w100
        stop <- "EinstellungenFertig" stop-if-true
        n65 = Wait (ms)(milliseconds to wait=u32 500 ("Zu wartende ms")) -> ()  [unwired: 1 out]
        n66 = case shown="True" "AIsNamenZurücksetzen" {
          frame False {
          }
          frame True {
            w206 = 32 ("Länge")
            w207 = string[] ["Mod1/AI0", "Mod1/AI1", "Mod1/AI2", "Mod1/AI3", "Mod1/AI4", "Mod1/AI5", "Mod1/AI6", "Mod1/AI7", "Mod1/AI8", "Mod1/AI9", "Mod1/AI10", "Mod1/AI11", "Mod1/AI12", "Mod1/AI13", "Mod1/AI14", "Mod1/AI15", "Mod1/AI16", "Mod1/AI17", "Mod1/AI18", "Mod1/AI19", "Mod1/AI20", "Mod1/AI21", "Mod1/AI22", "Mod1/AI23", "Mod1/AI24", "Mod1/AI25", "Mod1/AI26", "Mod1/AI27", "Mod1/AI28", "Mod1/AI29", "Mod1/AI30", "Mod1/AI31", "Mod2/AI0", "Mod2/AI1", "Mod2/AI2", "Mod2/AI3", "Mod2/AI4", "Mod2/AI5", "Mod2/AI6", "Mod2/AI7", "Mod2/AI8", "Mod2/AI9", "Mod2/AI10", "Mod2/AI11", "Mod2/AI12", "Mod2/AI13", "Mod2/AI14", "Mod2/AI15", "Mod2/AI16", "Mod2/AI17", "Mod2/AI18", "Mod2/AI19", "Mod2/AI20", "Mod2/AI21", "Mod2/AI22", "Mod2/AI23", "Mod2/AI24", "Mod2/AI25", "Mod2/AI26", "Mod2/AI27", "Mod2/AI28", "Mod2/AI29", "Mod2/AI30", "Mod2/AI31", "Mod3/AI0", "Mod3/AI1", "Mod3/AI2", "Mod3/AI3", "Mod3/AI4", "Mod3/AI5", "Mod3/AI6", "Mod3/AI7", "Mod3/AI8", "Mod3/AI9", "Mod3/AI10", "Mod3/AI11", "Mod3/AI12", "Mod3/AI13", "Mod3/AI14", "Mod3/AI15", "Mod3/AI16", "Mod3/AI17", "Mod3/AI18", "Mod3/AI19", "Mod3/AI20", "Mod3/AI21", "Mod3/AI22", "Mod3/AI23", "Mod3/AI24", "Mod3/AI25", "Mod3/AI26", "Mod3/AI27", "Mod3/AI28", "Mod3/AI29", "Mod3/AI30", "Mod3/AI31"] ("Array 2")
            n67 = Array Subset(array=w207, index=32 ("Index"), length=w206) -> (w203:string[])
            n68 = Array Subset(array=w207, index=0 ("Index"), length=w206) -> (w204:string[])
            n69 = Array Subset(array=w207, index=64 ("Index"), length=w206) -> (w202:string[])
            n70 = local write "Modul2/AIsNamen"(w203) -> ()
            n71 = local write "Modul1/AIsNamen"(w204) -> ()
            n72 = local write "Modul3/AIsNamen"(w202) -> ()
          }
        }
        n73 = Array Size(array="ReglerNameMod0") -> (size(s)=w190:i32)
        n74 = Array Size(array="ReglerNameMod1") -> (size(s)=w189:i32)
        n75 = Array Size(array="ReglerNameMod2A") -> (size(s)=w188:i32)
        n76 = Array Size(array="ReglerNameMod2B") -> (size(s)=w187:i32)
        n77 = Build Array "Anzahl Horst/Modul"(w190, w189, w188, w187) -> (w139:i32[])
        n78 = flat-sequence {
          tunnel: w139 -> [w200]
          tunnel: [w201] -> w138
          frame #0 {
            "AnzahlRegler/Modul" <- w200
          }
          frame #1 {
            n79 = local read "AnzahlRegler/Modul"() -> (w201:i32[])
          }
        }
        n80 = Build Array (concatenate)("Modul1/AIsNamen", "Modul2/AIsNamen", "Modul3/AIsNamen") -> (w140:string[])
        n81 = Bundle("DIOsMod0Nr"="DIOsMod0Nr", "DIOsMod1Nr"="DIOsMod1Nr", "DIOsMod2ANr"="DIOsMod2ANr", "DIOsMod2BNr"="DIOsMod2BNr", "AIsLH"="AIsLH", "AnzahlRegler/Modul"=w138, "Regler für den Probenfluß"="Regler für den Probenfluß", "SPvorgebenMod0"="SPvorgebenMod0", "SPvorgebenMod1"="SPvorgebenMod1", "SPvorgebenMod2A"="SPvorgebenMod2A", "SPvorgebenMod2B"="SPvorgebenMod2B", "MWAntwortMod0"="MWAntwortMod0", "MWAntwortMod1"="MWAntwortMod1", "MWAntwortMod2A"="MWAntwortMod2A", "MWAntwortMod2B"="MWAntwortMod2B", "FaktorMod0"="FaktorMod0", "FaktorMod1"="FaktorMod1", "FaktorMod2A"="FaktorMod2A", "FaktorMod2B"="FaktorMod2B", "MWabfragenMod0"="MWabfragenMod0", "MWabfragenMod1"="MWabfragenMod1", "MWabfragenMod2A"="MWabfragenMod2A", "MWabfragenMod2B"="MWabfragenMod2B", "Modul1/AI koeff"="Modul1/AI koeff", "Modul2/AI koeff"="Modul2/AI koeff", "Modul3/AI koeff"="Modul3/AI koeff", "Traps/MachsKoeff T(R)"="Traps/MachsKoeff T(R)", "Modul1/AIsNamen"="Modul1/AIsNamen", "Modul2/AIsNamen"="Modul2/AIsNamen", "Modul3/AIsNamen"="Modul3/AIsNamen", "DIOsMod0Name"="DIOsMod0Name", "DIOsMod1Name"="DIOsMod1Name", "DIOsMod2AName"="DIOsMod2AName", "DIOsMod2BName"="DIOsMod2BName", "ReglerNameMod0"="ReglerNameMod0", "ReglerNameMod1"="ReglerNameMod1", "ReglerNameMod2A"="ReglerNameMod2A", "ReglerNameMod2B"="ReglerNameMod2B", "Startmethode"="Startmethode", "Dateiordner Housekeeping"="Dateiordner Housekeeping", "Dateiname Housekeeping"="Dateiname Housekeeping", "DateiordnerECD1"="DateiordnerECD1", "DateinameECD1"="DateinameECD1", "DateiordnerECD2"="DateiordnerECD2", "DateinameECD2"="DateinameECD2", "LangsameHeizungen"="LangsameHeizungen", "ModuleLH"="ModuleLH", "Metavariablen"="Metavariablen", "Modul1/AI sicherer Bereich"="Modul1/AI sicherer Bereich", "Modul2/AI sicherer Bereich"="Modul2/AI sicherer Bereich", "Modul3/AI sicherer Bereich"="Modul3/AI sicherer Bereich", "Traps/Machs sicherer Bereich"="Traps/Machs sicherer Bereich", "ReglerMod0 sicherer Bereich"="ReglerMod0 sicherer Bereich", "ReglerMod1 sicherer Bereich"="ReglerMod1 sicherer Bereich", "ReglerMod2A sicherer Bereich"="ReglerMod2A sicherer Bereich", "ReglerMod2B sicherer Bereich"="ReglerMod2B sicherer Bereich", "Metavariablen grüner Bereich"="Metavariablen grüner Bereich", "Traps/MachsKoeff R(U)"="Traps/MachsKoeff R(U)", "LHGruppe"="LHGruppe") -> (w135:T8)  [unwired: 1 in]
        n82 = case shown="True" "EinstellungenSpeichern" {
          tunnel: w135 -> [_ w196]
          frame False {
          }
          frame True {
            n83 = Open/Create/Replace File(file path (use dialog)=path "c:/einstellungen.pery" ("Dateipfad Einstellungen"), operation (0:open)=T7."replace or create" ("Operation (0:Öffnen)")) -> (refnum out=w198:refnum<file>, error out=w195:errorcluster)  [unwired: 4 in, 1 out]
            n84 = Write to Binary File(file (use dialog)=w198, data=w196, error in=w195) -> (refnum out=w197:refnum<file>, error out=w194:errorcluster)  [unwired: 3 in, 1 out]
            n85 = Close File(refnum=w197, error in=w194) -> (error out=w193:errorcluster)  [unwired: 1 out]
            n86 = call <vilib>:"Simple Error Handler.vi"("error in (no error)"=w193) -> ()  [unwired: 4 in, 5 out]
          }
        }
      }
      n87 = Build Array (concatenate)(w109, w110, w111, w112) -> (w108:string[])
    }
    frame #2 {
      w225 = string[] ["<", "<=", "=", ">=", ">", "=/="] ("Strings []")
      n88 = for {
        tunnel: w220 -> [w332] mode=indexing
        tunnel: [w330] -> w219 mode=indexing
        n89 = Concatenate Strings(w332, " heizen?" ("String")) -> (w330:string)
      }
      n90 = Build Array (concatenate)(w232, w231, w230, w229) -> (w213:string[])
      n91 = Array Size(array=w213) -> (size(s)=w210:i32)
      n92 = for {
        tunnel: w212 -> [w250] mode=indexing
        tunnel: [w249] -> w211 mode=indexing
        tunnel: w210 -> [w248]
        n93 = Unbundle(w250) -> ("Zykluslängen [s]"=w303:dbl[], "ZeitpktDIOsMod0"=w302:dbl[], "ZeitpktDIOsMod1"=w301:dbl[], "ZeitpktDIOsMod2A"=w300:dbl[], "ZeitpktDIOsMod2B"=w299:dbl[], "DIOsSPMod0"=w298:bool[][], "DIOsSPMod1"=w297:bool[][], "DIOsSPMod2A"=w296:bool[][], "DIOsSPMod2B"=w295:bool[][], "Mod0HorstZeitpkt"=w294:dbl[], "Mod1HorstZeitpkt"=w293:dbl[], "Mod2AHorstZeitpkt"=w292:dbl[], "Mod2BHorstZeitpkt"=w291:dbl[], "HorstSPMod0"=w290:dbl[][], "HorstSPMod1"=w289:dbl[][], "HorstSPMod2A"=w288:dbl[][], "HorstSPMod2B"=w287:dbl[][], "LHSetpoints"=w286:dbl[], "LHHeizen?"=w285:bool[], "ZPktFPGABoolesch"=w284:dbl[], "FPGABoolesch"=w261:bool[][], "ZeitpktFPGAPID"=w283:dbl[], "ZeitpktFPGAFixp"=w281:dbl[], "SHSetpoints"=w256:dbl[][], "t_PreMach1"=w280:dbl[], "T_PreMach1"=w279:dbl[], "t_PreMach2"=w278:dbl[], "T_PreMach2"=w277:dbl[], "PIDs für \"träge\" Heizungen"=w276:T9, "Zwangsbedingungen"=w247:dbl[][], "Dateien fürs MS schicken?"=w275:bool, "ZeitpunkteMPV"=w274:dbl[], "SPMPV"=w273:i32[], "ZeitpktMS-1"=w272:dbl, "ZeitpktMS-2"=w271:dbl, "Int.Start1"=w270:dbl, "Int.Stop1"=w269:dbl, "Int.Start2"=w268:dbl, "Int.Stop2"=w267:dbl, "Methodenname"=w266:string, "t_MainMach1"=w265:dbl[], "T_MainMach1"=w264:dbl[], "t_MainMach2"=w263:dbl[], "T_MainMach2"=w262:dbl[])  [unwired: 1 out]
        n94 = for {
          tunnel: w247 -> [w315] mode=indexing
          tunnel: w248 -> [w318]
          tunnel: [w314] -> w246 mode=indexing
          tunnel: [w308] -> w245 mode=indexing
          i -> [w310]
          n95 = Add(x=w318, y=3) -> (x+y=w317:i32)
          n96 = Index Array(array=w315, index=6) -> (element=w316:dbl)
          n97 = To Double Precision Float(number=w317) -> (double precision float=w320:dbl)
          n98 = Greater?(x=w316, y=w320) -> (0:w319:bool)
          n99 = case shown="False" w319 {
            tunnel: w315 -> [w323 w329]
            tunnel: w316 -> [_ w326]
            tunnel: [w323 w324] -> w314
            frame False {
            }
            frame True {
              n100 = Subtract(x=w326, y=4.0) -> (x-y=w327:dbl)
              n101 = Replace Array Subset(array=w329, new element=w327, index=6) -> (w324:dbl[])
            }
          }
          n102 = Greater Or Equal?(x=w316, y=w318) -> (x >= y?=w313:bool)
          n103 = Less Or Equal?(x=w316, y=w317) -> (x <= y?=w312:bool)
          n104 = And(x=w313, y=w312) -> (x .and. y?=w311:bool)
          n105 = Select(t=w310, s=w311, f=-1) -> (s? t:f=w308:i32)
        }
        n106 = Index Array(array=w256, index (col) #1=0 ("disabled index (col)"), index (col) #2=2 ("index (col)")) -> (element #1=w254:dbl[], element #2=w253:dbl[])  [unwired: 2 in]
        n107 = Delete From Array(array=w261, length=4, index (col)=0 ("disabled index (col)")) -> (array with subset deleted=w258:bool[][])  [unwired: 1 in, 1 out]
        n108 = Build Array(w254, w253) -> (w252:dbl[][])
        n109 = Transpose 2D Array(2D array=w252) -> (transposed array=w251:dbl[][])
        n110 = Reverse 1D Array(array=w245) -> (reversed array=w244:i32[])
        n111 = for {
          tunnel: w244 -> [w305] mode=indexing
          shift-right: [w304] -> w243
          shift-left: w246 -> [w307]
          n112 = Delete From Array(array=w307, length=1, index (row)=w305) -> (array with subset deleted=w304:dbl[][])  [unwired: 1 in, 1 out]
        }
        n113 = Bundle("Zykluslängen [s]"=w303, "ZeitpktDIOsMod0"=w302, "ZeitpktDIOsMod1"=w301, "ZeitpktDIOsMod2A"=w300, "ZeitpktDIOsMod2B"=w299, "DIOsSPMod0"=w298, "DIOsSPMod1"=w297, "DIOsSPMod2A"=w296, "DIOsSPMod2B"=w295, "Mod0HorstZeitpkt"=w294, "Mod1HorstZeitpkt"=w293, "Mod2AHorstZeitpkt"=w292, "Mod2BHorstZeitpkt"=w291, "HorstSPMod0"=w290, "HorstSPMod1"=w289, "HorstSPMod2A"=w288, "HorstSPMod2B"=w287, "LHSetpoints"=w286, "LHHeizen?"=w285, "ZPktFPGABoolesch"=w284, "FPGABoolesch"=w258, "ZeitpktFPGAPID"=w283, "FPGAPID"=T4 [], "ZeitpktFPGAFixp"=w281, w251, "t_PreMach1"=w280, "T_PreMach1"=w279, "t_PreMach2"=w278, "T_PreMach2"=w277, "PIDs für \"träge\" Heizungen"=w276, "Zwangsbedingungen"=w243, "Dateien fürs MS schicken?"=w275, "ZeitpunkteMPV"=w274, "SPMPV"=w273, "ZeitpktMS-1"=w272, "ZeitpktMS-2"=w271, "Int.Start1"=w270, "Int.Stop1"=w269, "Int.Start2"=w268, "Int.Stop2"=w267, "Methodenname"=w266, "t_MainMach1"=w265, "T_MainMach1"=w264, "t_MainMach2"=w263, "T_MainMach2"=w262) -> (w249:T10)  [unwired: 1 in]
      }
      n114 = Build Array (concatenate)(w213, string[] ["Heizen?Trap1", "Heizen?Trap2", "Heizen?PreMach1", "Heizen?PreMach2", "Heizen?MainMach1", "Heizen?MainMach2", "Methodennummer", "STOPP!!!"], w219, w221, "PositionMPV", w216) -> (w227:string[])
      n115 = Build Array (concatenate)(w234, string[] ["T-Trap1", "T-Trap2", "T-PreMach1", "T-PreMach2", "T-MainMach1", "T-MainMach2"], w221, string[] ["Gesamte Zeit", "Methodenzeit", "Zykluszeit Mod0", "Zykluszeit Mod1", "Zykluszeit Mod2A", "Zykluszeit Mod2B"] ("Array"), "PositionMPV", w218) -> (w226:string[])
      n116 = property on="Vergleichsoperator2" class="Ring (strikt)"("Strings []"=w225) -> ()  [unwired: 2 in, 2 out]
      n117 = while {
        tunnel: w242 -> [w401]
        tunnel: w241 -> [w400]
        tunnel: w240 -> [w399]
        tunnel: w239 -> [w398]
        tunnel: w238 -> [w397]
        tunnel: w237 -> [w396]
        tunnel: w236 -> [w395]
        tunnel: w235 -> [w394]
        shift-right: [w354] -> w214
        shift-left: w211 -> [w336]
        tunnel: w226 -> [w361]
        tunnel: w225 -> [w360]
        tunnel: w227 -> [w359]
        tunnel: w223 -> [w353]
        stop <- w391 stop-if-true
        n118 = Index Array(array=w336, index="Methode Nummer") -> (element=w390:T10)
        n119 = Unbundle(w390) -> ("Zykluslängen [s]"=w389:dbl[], "ZeitpktDIOsMod0"=w388:dbl[], "ZeitpktDIOsMod1"=w387:dbl[], "ZeitpktDIOsMod2A"=w386:dbl[], "ZeitpktDIOsMod2B"=w385:dbl[], "DIOsSPMod0"=w384:bool[][], "DIOsSPMod1"=w383:bool[][], "DIOsSPMod2A"=w382:bool[][], "DIOsSPMod2B"=w381:bool[][], "Mod0HorstZeitpkt"=w380:dbl[], "Mod1HorstZeitpkt"=w379:dbl[], "Mod2AHorstZeitpkt"=w378:dbl[], "Mod2BHorstZeitpkt"=w377:dbl[], "HorstSPMod0"=w376:dbl[][], "HorstSPMod1"=w375:dbl[][], "HorstSPMod2A"=w374:dbl[][], "HorstSPMod2B"=w373:dbl[][], "LHSetpoints"=w372:dbl[], "LHHeizen?"=w371:bool[], "ZPktFPGABoolesch"=w370:dbl[], "FPGABoolesch"=w369:bool[][], "ZeitpktFPGAPID"=w368:dbl[], "FPGAPID"=w333:T4, "ZeitpktFPGAFixp"=w367:dbl[], w366:dbl[][], "t_PreMach1"=w365:dbl[], "T_PreMach1"=w364:dbl[], "t_PreMach2"=w363:dbl[], "T_PreMach2"=w362:dbl[], "PIDs für \"träge\" Heizungen"=w358:T9, "Zwangsbedingungen"=w357:dbl[][], "Dateien fürs MS schicken?"=w356:bool, "ZeitpunkteMPV"=w349:dbl[], "SPMPV"=w348:i32[], "ZeitpktMS-1"=w351:dbl, "ZeitpktMS-2"=w350:dbl, "Int.Start1"=w347:dbl, "Int.Stop1"=w346:dbl, "Int.Start2"=w345:dbl, "Int.Stop2"=w344:dbl, "Methodenname"=w352:string, "t_MainMach1"=w343:dbl[], "T_MainMach1"=w342:dbl[], "t_MainMach2"=w341:dbl[], "T_MainMach2"=w340:dbl[])
        n120 = property on="LHHeizen?" class="Arr (strikt)"("Value"=w371) -> ()  [unwired: 2 in, 2 out]
        n121 = property on="FPGAPID" class="Arr (strikt)"("Value"=w333) -> ()  [unwired: 2 in, 2 out]
        n122 = property on="SPMPV" class="Arr (strikt)"("Value"=w348) -> ()  [unwired: 2 in, 2 out]
        n123 = property on="Int.Start1" class="DigWert (strikt)"("Value"=w347) -> ()  [unwired: 2 in, 2 out]
        n124 = property on="Int.Stop1" class="DigWert (strikt)"("Value"=w346) -> ()  [unwired: 2 in, 2 out]
        n125 = property on="Int.Start2" class="DigWert (strikt)"("Value"=w345) -> ()  [unwired: 2 in, 2 out]
        n126 = property on="Int.Stop2" class="DigWert (strikt)"("Value"=w344) -> ()  [unwired: 2 in, 2 out]
        n127 = property on="T_MainMach2" class="Arr (strikt)"("Value"=w340) -> ()  [unwired: 2 in, 2 out]
        n128 = property on="Zykluslängen [s]" class="Arr (strikt)"("Value"=w389) -> ()  [unwired: 2 in, 2 out]
        n129 = property on="ZeitpktDIOsMod0" class="Arr (strikt)"("Value"=w388) -> ()  [unwired: 2 in, 2 out]
        n130 = property on="Mod2BHorstZeitpkt" class="Arr (strikt)"("Value"=w377) -> ()  [unwired: 2 in, 2 out]
        n131 = property on="HorstSPMod0" class="Arr (strikt)"("Value"=w376) -> ()  [unwired: 2 in, 2 out]
        n132 = property on="LHSetpoints" class="Arr (strikt)"("Value"=w372) -> ()  [unwired: 2 in, 2 out]
        n133 = property on="ZPktFPGABoolesch" class="Arr (strikt)"("Value"=w370) -> ()  [unwired: 2 in, 2 out]
        n134 = property on="FPGABoolesch" class="Arr (strikt)"("Value"=w369) -> ()  [unwired: 2 in, 2 out]
        n135 = property on="T_PreMach2" class="Arr (strikt)"("Value"=w362) -> ()  [unwired: 2 in, 2 out]
        n136 = property on="PIDs für \"träge\" Heizungen" class="Arr (strikt)"("Value"=w358) -> ()  [unwired: 2 in, 2 out]
        n137 = while {
          tunnel: w400 -> [w509]
          tunnel: w399 -> [w508]
          tunnel: w398 -> [w507]
          tunnel: w397 -> [w506]
          tunnel: w396 -> [w505]
          tunnel: w394 -> [w504]
          tunnel: w395 -> [w503]
          tunnel: w401 -> [w473]
          tunnel: [w472] -> w392
          tunnel: [w435] -> w393
          tunnel: ["EditorBeenden"] -> w391
          tunnel: w361 -> [w458]
          shift-right: [w453] -> _
          shift-left: w357 -> [w457]
          tunnel: w360 -> [w456]
          tunnel: w359 -> [w455]
          tunnel: ["AllesSpeichern"] -> w355
          tunnel: ["MethodeDuplizieren"] -> w338
          stop <- w427 stop-if-true
          n138 = for {
            tunnel: w457 -> [w518] mode=indexing
            tunnel: w458 -> [w514]
            tunnel: w456 -> [w513]
            tunnel: w455 -> [w532]
            tunnel: [w526] -> w466 mode=indexing
            n139 = Index Array(array=w518, index=0 ("Index")) -> (element=w538:dbl)
            n140 = Index Array(array=w518, index=1 ("Index")) -> (element=w536:dbl)
            n141 = Index Array(array=w518, index=3 ("Index")) -> (element=w520:dbl)
            n142 = Index Array(array=w518, index=4 ("Index")) -> (element=w519:dbl)
            n143 = Index Array(array=w518, index=6 ("Index")) -> (element=w534:dbl)
            n144 = To Long Integer(number=w538) -> (32bit integer=w537:i32)
            n145 = To Long Integer(number=w536) -> (32bit integer=w535:i32)
            n146 = To Long Integer(number=w520) -> (32bit integer=w517:i32)
            n147 = To Long Integer(number=w519) -> (32bit integer=w516:i32)
            n148 = To Long Integer(number=w534) -> (32bit integer=w533:i32)
            n149 = Index Array(array=w518, index=2 ("Index")) -> (element=w531:dbl)
            n150 = Index Array(array=w518, index=5 ("Index")) -> (element=w515:dbl)
            n151 = Index Array(array=w518, index=7 ("Index")) -> (element=w530:dbl)
            n152 = Index Array(array=w514, index=w537) -> (element=w529:string)
            n153 = Index Array(array=w513, index=w535) -> (element=w528:string)
            n154 = Index Array(array=w514, index=w517) -> (element=w512:string)
            n155 = Index Array(array=w513, index=w516) -> (element=w511:string)
            n156 = Index Array(array=w532, index=w533) -> (element=w524:string)
            n157 = Number To Exponential String(number=w531) -> (E-format string=w527:string)  [unwired: 3 in]
            n158 = Number To Exponential String(number=w515) -> (E-format string=w510:string)  [unwired: 3 in]
            n159 = Number To Exponential String(number=w530) -> (E-format string=w525:string)  [unwired: 3 in]
            n160 = Build Array(w529, w528, w527, w512, w511, w510, w524, w525) -> (w526:string[])
          }
          "ZwangsBedingungen" <- w466
          n161 = Wait (ms)(milliseconds to wait=u32 500 ("Zu wartende ms")) -> ()  [unwired: 1 out]
          n162 = Build Array("AbfragbareVariablen1", "Vergleichsoperator1", "Wert1", "AbfragbareVariablen2", "Vergleichsoperator2", "Wert2", "BedienbareVariablen", "Ausgangswert") -> (w463:dbl[])
          n163 = case shown="False" "Bedingung übernehmen" {
            tunnel: w457 -> [w548 w551]
            tunnel: w463 -> [_ w550]
            tunnel: [w548 w549] -> w464
            frame False {
            }
            frame True {
              n164 = Build Array (concatenate)(w551, w550) -> (w549:dbl[][])
            }
          }
          n165 = case shown="True" "löschen" {
            tunnel: w464 -> [w544 w547]
            tunnel: [w544 w545] -> w453
            frame False {
            }
            frame True {
              n166 = Delete From Array(array=w547, index (row)="Bedingung Nr. X") -> (array with subset deleted=w545:dbl[][])  [unwired: 2 in, 1 out]
            }
          }
          n167 = Or(x="MethodeSpeichern", y="EditorBeenden") -> (x .or. y?=w470:bool)
          n168 = Or(x=w470, y="MethodeLaden") -> (x .or. y?=w437:bool)
          n169 = local write "Zwangsbedingungen"(w453) -> ()
          n170 = Or(x=w437, y="AllesSpeichern") -> (x .or. y?=w428:bool)
          n171 = Or(x="MethodeDuplizieren", y=w428) -> (x .or. y?=w427:bool)
          n172 = Or(x="AllesSpeichern", y="MethodeSpeichern") -> (x .or. y?=w435:bool)
          n173 = Bundle("Zykluslängen [s]"="Zykluslängen [s]", "ZeitpktDIOsMod0"="ZeitpktDIOsMod0", "ZeitpktDIOsMod1"="ZeitpktDIOsMod1", "ZeitpktDIOsMod2A"="ZeitpktDIOsMod2A", "ZeitpktDIOsMod2B"="ZeitpktDIOsMod2B", "DIOsSPMod0"="DIOsSPMod0", "DIOsSPMod1"="DIOsSPMod1", "DIOsSPMod2A"="DIOsSPMod2A", "DIOsSPMod2B"="DIOsSPMod2B", "Mod0HorstZeitpkt"="Mod0HorstZeitpkt", "Mod1HorstZeitpkt"="Mod1HorstZeitpkt", "Mod2AHorstZeitpkt"="Mod2AHorstZeitpkt", "Mod2BHorstZeitpkt"="Mod2BHorstZeitpkt", "HorstSPMod0"="HorstSPMod0", "HorstSPMod1"="HorstSPMod1", "HorstSPMod2A"="HorstSPMod2A", "HorstSPMod2B"="HorstSPMod2B", "LHSetpoints"="LHSetpoints", "LHHeizen?"="LHHeizen?", "ZPktFPGABoolesch"="ZPktFPGABoolesch", "FPGABoolesch"="FPGABoolesch", "ZeitpktFPGAPID"="ZeitpktFPGAPID", "FPGAPID"="FPGAPID", "ZeitpktFPGAFixp"="ZeitpktFPGAFixp", "SHSetpoints"="SHSetpoints", "t_PreMach1"="t_PreMach1", "T_PreMach1"="T_PreMach1", "t_PreMach2"="t_PreMach2", "T_PreMach2"="T_PreMach2", "PIDs für \"träge\" Heizungen"="PIDs für \"träge\" Heizungen", "Zwangsbedingungen"="Zwangsbedingungen", "Dateien fürs MS schicken?"="Dateien fürs MS schicken?", "ZeitpunkteMPV"="ZeitpunkteMPV", "SPMPV"="SPMPV", "ZeitpktMS-1"="ZeitpktMS-1", "ZeitpktMS-2"="ZeitpktMS-2", "Int.Start1"="Int.Start1", "Int.Stop1"="Int.Stop1", "Int.Start2"="Int.Start2", "Int.Stop2"="Int.Stop2", "Methodenname"="Methodenname", "t_MainMach1"="t_MainMach1", "T_MainMach1"="T_MainMach1", "t_MainMach2"="t_MainMach2", "T_MainMach2"="T_MainMach2") -> (w472:T11)  [unwired: 1 in]
          "DIOsMod0Name" <- w473
          "DIOsMod1Name" <- w509
          "DIOsMod2AName" <- w508
          "DIOsMod2BName" <- w507
          "HorstMod0Name" <- w506
          "HorstMod2BName" <- w503
          "HorstMod2AName" <- w504
          "HorstMod1Name" <- w505
        }
        n174 = property on="DIOsSPMod1" class="Arr (strikt)"("Value"=w383) -> ()  [unwired: 2 in, 2 out]
        n175 = property on="DIOsSPMod2A" class="Arr (strikt)"("Value"=w382) -> ()  [unwired: 2 in, 2 out]
        n176 = property on="HorstSPMod1" class="Arr (strikt)"("Value"=w375) -> ()  [unwired: 2 in, 2 out]
        n177 = property on="HorstSPMod2A" class="Arr (strikt)"("Value"=w374) -> ()  [unwired: 2 in, 2 out]
        n178 = property on="HorstSPMod2B" class="Arr (strikt)"("Value"=w373) -> ()  [unwired: 2 in, 2 out]
        n179 = property on="ZeitpktFPGAPID" class="Arr (strikt)"("Value"=w368) -> ()  [unwired: 2 in, 2 out]
        n180 = property on="ZeitpktFPGAFixp" class="Arr (strikt)"("Value"=w367) -> ()  [unwired: 2 in, 2 out]
        n181 = property on="SHSetpoints" class="Arr (strikt)"("Value"=w366) -> ()  [unwired: 2 in, 2 out]
        n182 = property on="t_PreMach1" class="Arr (strikt)"("Value"=w365) -> ()  [unwired: 2 in, 2 out]
        n183 = property on="T_PreMach1" class="Arr (strikt)"("Value"=w364) -> ()  [unwired: 2 in, 2 out]
        n184 = property on="t_PreMach2" class="Arr (strikt)"("Value"=w363) -> ()  [unwired: 2 in, 2 out]
        n185 = property on="ZeitpktDIOsMod1" class="Arr (strikt)"("Value"=w387) -> ()  [unwired: 2 in, 2 out]
        n186 = property on="ZeitpktDIOsMod2A" class="Arr (strikt)"("Value"=w386) -> ()  [unwired: 2 in, 2 out]
        n187 = property on="ZeitpktDIOsMod2B" class="Arr (strikt)"("Value"=w385) -> ()  [unwired: 2 in, 2 out]
        n188 = property on="DIOsSPMod0" class="Arr (strikt)"("Value"=w384) -> ()  [unwired: 2 in, 2 out]
        n189 = property on="DIOsSPMod2B" class="Arr (strikt)"("Value"=w381) -> ()  [unwired: 2 in, 2 out]
        n190 = property on="Mod0HorstZeitpkt" class="Arr (strikt)"("Value"=w380) -> ()  [unwired: 2 in, 2 out]
        n191 = property on="Mod1HorstZeitpkt" class="Arr (strikt)"("Value"=w379) -> ()  [unwired: 2 in, 2 out]
        n192 = property on="Mod2AHorstZeitpkt" class="Arr (strikt)"("Value"=w378) -> ()  [unwired: 2 in, 2 out]
        n193 = property on="Dateien fürs MS schicken?" class="Bool. (strikt)"("Value"=w356) -> ()  [unwired: 2 in, 2 out]
        n194 = property on="ZeitpunkteMPV" class="Arr (strikt)"("Value"=w349) -> ()  [unwired: 2 in, 2 out]
        n195 = property on="ZeitpktMS-1" class="DigWert (strikt)"("Value"=w351) -> ()  [unwired: 2 in, 2 out]
        n196 = property on="ZeitpktMS-2" class="DigWert (strikt)"("Value"=w350) -> ()  [unwired: 2 in, 2 out]
        n197 = property on="Methodenname" class="Str"("Value"=w352) -> ()  [unwired: 2 in, 2 out]
        n198 = property on="t_MainMach1" class="Arr (strikt)"("Value"=w343) -> ()  [unwired: 2 in, 2 out]
        n199 = property on="T_MainMach1" class="Arr (strikt)"("Value"=w342) -> ()  [unwired: 2 in, 2 out]
        n200 = property on="t_MainMach2" class="Arr (strikt)"("Value"=w341) -> ()  [unwired: 2 in, 2 out]
        n201 = case shown="True" "MethodeLöschen" {
          tunnel: w336 -> [w402 w406]
          tunnel: [w402 w403] -> w335
          tunnel: "Methode Nummer" -> [_ w404]
          frame False {
          }
          frame True {
            n202 = invoke on="MethodeLöschen" class="Bool (strict)" method="Std wiederherstellen"() -> ()  [unwired: 3 in, 3 out]
            n203 = Delete From Array(array=w406, length=1, index=w404) -> (array with subset deleted=w403:T12)  [unwired: 1 out]
          }
        }
        n204 = case shown="True" w338 {
          tunnel: w335 -> [w407 w410]
          tunnel: [w407 w409] -> w339
          tunnel: "Methode Nummer" -> [_ w411]
          frame False {
          }
          frame True {
            n205 = Index Array(array=w410, index=w411) -> (element=w408:T10)
            n206 = Build Array (concatenate)(w410, w408) -> (w409:T12)
          }
        }
        n207 = case shown="True" w393 {
          tunnel: w339 -> [w420 w426]
          tunnel: w392 -> [_ w421]
          tunnel: [w420 w422] -> w354
          tunnel: "Methode Nummer" -> [_ w423]
          frame False {
          }
          frame True {
            n208 = Delete From Array(array=w426, length=1 ("Länge"), index=w423) -> (array with subset deleted=w424:T12)  [unwired: 1 out]
            n209 = Insert Into Array(array=w424, index=w423, new element=w421) -> (w422:T12)
          }
        }
        n210 = case shown="True" w355 {
          tunnel: w354 -> [_ w417]
          tunnel: w353 -> [_ w412]
          frame False {
          }
          frame True {
            n211 = Open/Create/Replace File(file path (use dialog)=w412, operation (0:open)=T7."replace or create" ("Operation (0:Öffnen)")) -> (refnum out=w416:refnum<file>, error out=w418:errorcluster)  [unwired: 4 in, 1 out]
            n212 = Write to Binary File(file (use dialog)=w416, data=w417, error in=w418) -> (refnum out=w414:refnum<file>, error out=w415:errorcluster)  [unwired: 3 in, 1 out]
            n213 = Close File(refnum=w414, error in=w415) -> (error out=w413:errorcluster)  [unwired: 1 out]
            n214 = call <vilib>:"Simple Error Handler.vi"("error in (no error)"=w413) -> ()  [unwired: 4 in, 5 out]
          }
        }
      }
      "Methoden" <- w214
      n215 = property on="BedienbareVariablen" class="Ring (strikt)"("Strings []"=w227) -> ()  [unwired: 2 in, 2 out]
      n216 = property on="AbfragbareVariablen1" class="Ring (strikt)"("Strings []"=w226) -> ()  [unwired: 2 in, 2 out]
      n217 = property on="AbfragbareVariablen2" class="Ring (strikt)"("Strings []"=w226) -> ()  [unwired: 2 in, 2 out]
      n218 = property on="Vergleichsoperator1" class="Ring (strikt)"("Strings []"=w225) -> ()  [unwired: 2 in, 2 out]
      "LangsameHeizungen" <- w224
    }
  }
  n219 = call <vilib>:"Simple Error Handler.vi"("error in (no error)"=w20) -> ()  [unwired: 4 in, 5 out]
  n220 = Open/Create/Replace File(file path (use dialog)=path "C:/methoden.per" ("Dateipfad Methoden")) -> (refnum out=w18:refnum<file>, error out=w17:errorcluster)  [unwired: 5 in, 1 out]
  n221 = Read from Binary File(5:T6 [], 8:w17, 11:w18) -> (0:w15:errorcluster, 2:w6:T6, 3:w16:refnum<file>)  [unwired: 3 in, 1 out]
  n222 = Close File(refnum=w16, error in=w15) -> (path=w5:path, error out=w14:errorcluster)
  n223 = call <vilib>:"Simple Error Handler.vi"("error in (no error)"=w14) -> ()  [unwired: 4 in, 5 out]
  n224 = Path To String(path=w5) -> (string=w4:string)
  n225 = Concatenate Strings(w4, "y" ("string")) -> (w2:string)
  n226 = String To Path(string=w2) -> (path=w1:path)
